vi "Autopatch-v2.4_openlooop.vi"() -> ()   [LabVIEW 2018]
uses:
  <vilib>/userdefined/High Color/IMAQdx.ctl
  <vilib>/DAQmx/write.llb/DAQmx Write (Analog DBL 1Chan 1Samp).vi
  <vilib>/DAQmx/write.llb/DAQmx Write (Analog Wfm 1Chan NSamp).vi
  <vilib>/DAQmx/read.llb/DAQmx Read (Analog Wfm 1Chan NSamp).vi
  <vilib>/Analysis/baseanly.llb/Mean (DBL).vi
  <vilib>/DAQmx/create/channels.llb/DAQmx Create Channel (AO-Voltage-Basic).vi
  <vilib>/DAQmx/miscellaneous.llb/DAQmx Fill In Error Info.vi
  <vilib>/DAQmx/create/channels.llb/DAQmx Create Channel (AI-Voltage-Basic).vi
  <vilib>/DAQmx/configure/timing.llb/DAQmx Timing (Sample Clock).vi
  <vilib>/DAQmx/configure/trigger.llb/DAQmx Start Trigger (Digital Edge).vi
  <vilib>/Waveform/WDTOps.llb/WDT Waveform Duration DBL.vi
  <vilib>/addons/control/pid/pid.llb/PID (DBL).vi
  <vilib>/vision/driver/NI_Vision_Acquisition_Software.lvlib
  <resource>/objmgr/daqmx.rc
  <vilib>/Analysis/NI_AALBase.lvlib
  <vilib>/measure/NI_MABase.lvlib
  <vilib>/vision/NI_Vision_Development_Module.lvlib
  <vilib>/addons/control/pid/NI_PID_pid.lvlib
  <vilib>/Analysis/NI_AALPro.lvlib
panel:
  in  "傅里叶mp285下降步伐":dbl
  in  "下降40倍物镜状态机":u16(ring) items=["下降40倍物镜初始", "下降40倍物镜循环", "下降40倍物镜一段距离", "下降40倍物镜结束", ""]
  in  "气压选择":u16(ring) items=["高正压", "低正压", "大气压", "低负压", "高负压"]
  out "裁剪数组":i32[](array[numeric])
  out "自动接触状态":i32
  in  "没有细胞":bool=TRUE
  out "已发送图像":bool
  in  "发送次数":dbl
  in  "目标细胞位置":bool=TRUE
  out "错误输出 2":errorcluster caption="错误输出"
  out "Matches 2":T1(array[cluster]) {"Bounding Box"."y" format="%.2f"; "Bounding Box"."x" format="%.2f"; "Position"."y" format="%.2f"; "Position"."x" format="%.2f"; "Score" format="%.2f"; "Scale" format="%.2f"; "Angle" format="%.2f"}
  in  "基路径40":path=path "D:/韩宇/程序/CCD/模板40倍.jpg"
  out "傅里叶最大值":dbl
  out "傅里叶数组":bool[](array[boolean])
  in  "傅里叶状态机":u16(ring) items=["傅里叶初始", "傅里叶循环", "傅里叶暂停", "傅里叶结束"]
  out "图像检测到":bool=TRUE
  out "自动封接开始时间":u32
  out "针下降次数":i32
  in  "自动测试":bool
  in  "图像检测":bool
  out "写入的字节":i32
  out "数据输出 3":string
  out "X 3":i32
  out "Y 3":i32
  out "error IO":errorcluster
  out "Y 2":i32
  out "X 2":i32
  in  "开环移动针尖":bool
  in  "傅里叶":bool
  in  "下降物镜":bool
  in  "电极入液":bool
  out "自动接触初始":i32
  in  "枚举":enum16{"200ms", "500ms", "1000ms", ""}(ring)=enum."1000ms"
  out "dX/dt":dbl[](array[numeric])
  in  "下降/向右":bool
  in  "钳制电位":i16(ring) items=["0mv", "-70mv"]
  out "起始破膜时间":u32
  in  "自动破膜":bool
  in  "控制箱刺激ON\n/放大器刺激":bool=TRUE
  in  "自动封接":bool
  in  "保存数据":bool
  out "没匹配到？":bool
  in  "PID gains":T2={"proportional gain (Kc)"=-0.05, "integral time (Ti, min)"=0.0, "derivative time (Td, min)"=0.0} caption="PID增益" {"derivative time (Td, min)" format="%.3f"; "integral time (Ti, min)" format="%.3f"; "proportional gain (Kc)" format="%.3f"}
  in  "PID gains 2":T2={"proportional gain (Kc)"=0.05, "integral time (Ti, min)"=0.0, "derivative time (Td, min)"=0.0} caption="PID增益" {"derivative time (Td, min)" format="%.3f"; "integral time (Ti, min)" format="%.3f"; "proportional gain (Kc)" format="%.3f"}
  in  "下降步伐/um":dbl=1.0
  in  "自动接触":bool
  out "傅里叶求和":sgl(graph)
  in  "针尖移动":bool
  out "目标坐标":i32[](array[numeric])
  in  "针尖模板匹配":bool=TRUE
  in  "基路径20":path=path "D:/韩宇/程序/CCD/针尖水上模板4X.jpg"
  out "Number of Matches":i32
  in  "Minimum Contrast":i32 min=0 max=255 step=1
  in  "Minimum Match Score":sgl=500.0 min=0 max=1000 format="%.2f"
  in  "Number of Matches Requested":i32=1 min=1
  in  "Match Mode":u16(ring) items=["Shift Invariant", "Rotation Invariant"]
  out "针尖坐标":sgl[](array[numeric])
  out "校准的入液阻值":dbl
  out "错误输出 3":errorcluster caption="错误输出"
  out "测量值":dbl
  out "给定值":dbl
  out "输出气压波形图表":cluster{dbl, "低负":dbl}(graph)
  in  "低负":sgl(knob)=-0.45548448
  in  "高负":sgl(knob)=-5.0
  in  "低正":sgl(knob)=0.49642125 scale=0.0..2.0
  in  "高正":sgl(knob)=10.718505 scale=0.0..15.0
  in  "采样率":u32=255
  in  "DevIndex":i32
  in  "Holding Voltage":dbl=-70.0
  out "Negative Peak":dbl
  out "阻值波形图表":dbl(graph)
  out "Resistance(MΩ)":dbl
  out "！":bool
  in  "电压钳/电流钳":u16(ring) items=["Voltage Clamp", "Current Clamp"]
  out "电流信号波形图":waveform(dbl)(graph)
  in  "frequency":dbl=20.0
  in  "Averaging":i32=5
  in  "amplitude":dbl=0.01
  in  "阻值数组":dbl[](array[numeric])
  out "循环时间":u32
  out "Image":T3(plugin-control)
  in  "停止":bool
  in  "Session In":T4="cam1"
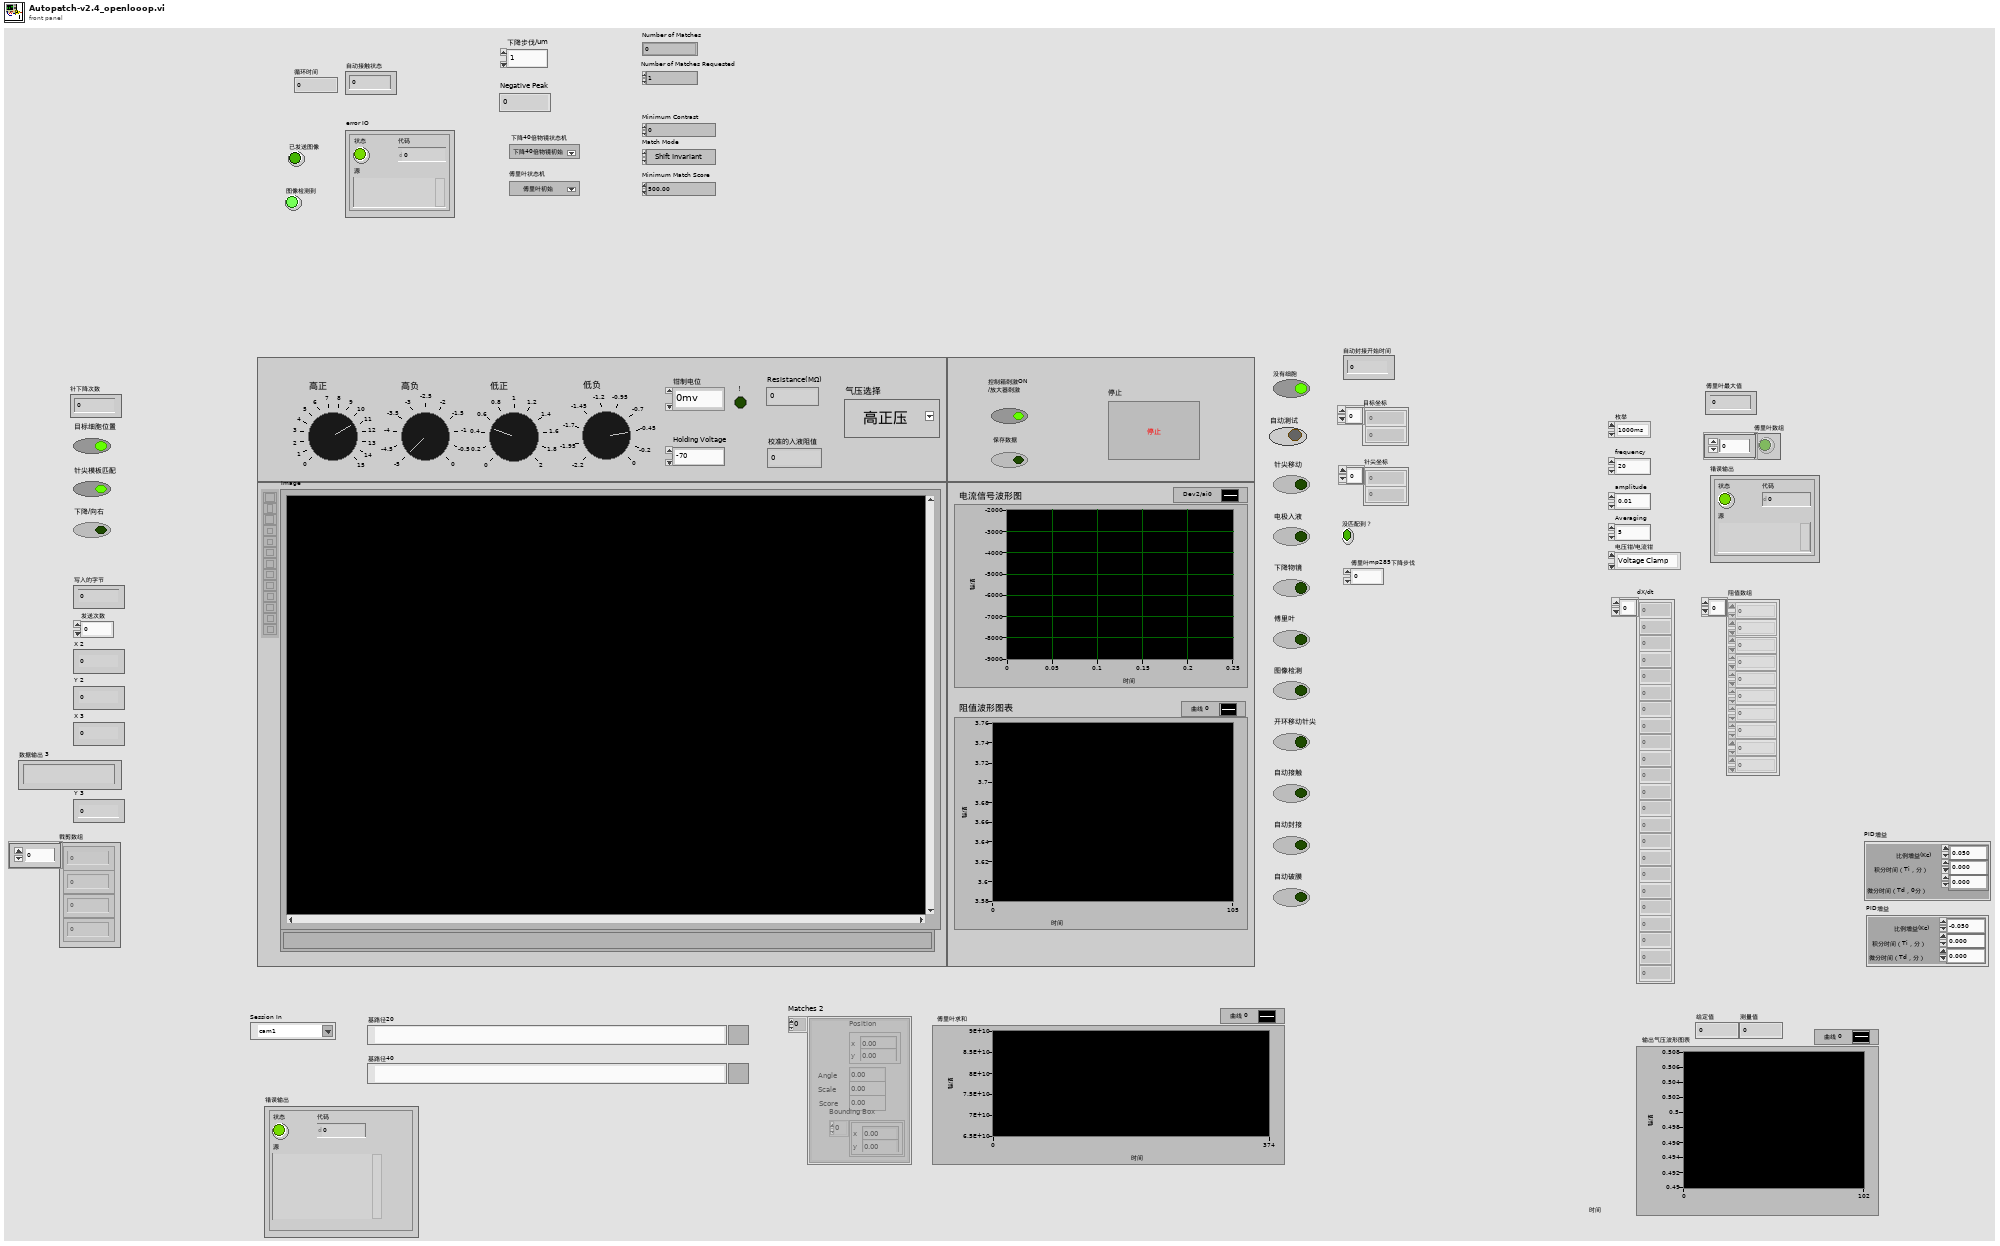
[diagram p1: front panel]
types:
  T1 = cluster{"Position":cluster{"x":sgl, "y":sgl}, "Angle":sgl, "Scale":sgl, "Score":sgl, "Bounding Box":cluster{"x":sgl, "y":sgl}[]}[]
  T2 = cluster{"proportional gain (Kc)":dbl, "integral time (Ti, min)":dbl, "derivative time (Td, min)":dbl}
  T3 = typedef "IMAQ Image.ctl" = refnum<image>
  T4 = typedef "IMAQdx.ctl" = refnum<k21>
  T5 = typedef "Image Type" = u32
  T6 = enum16{"open", "replace", "create", "open or create", "replace or create", "replace or create with confirmation"}
  T7 = cluster{"Averaging":i32, "frequency":dbl, "amplitude":dbl, "Proportion":dbl, "Fs":dbl}
  T8 = enum16{"Sine Wave", "Triangle Wave", "Square Wave", "Sawtooth Wave"}
  T9 = cluster{"Position":cluster{"x":sgl, "y":sgl}, "Angle":sgl, "Scale":sgl, "Score":sgl, "Bounding Box":cluster{"x":sgl, "y":sgl}[]}
  T10 = enum32{"Real", "Imaginary", "Magnitude", "Phase"}
  T11 = cluster{"Global Rectangle":i32[], "Contours":cluster{"Contour Type":u32, "ROI Type":u32, "Points":i32[]}[]}
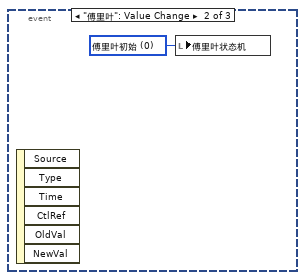
[diagram p7: hidden frame]
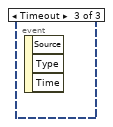
[diagram p8: hidden frame]
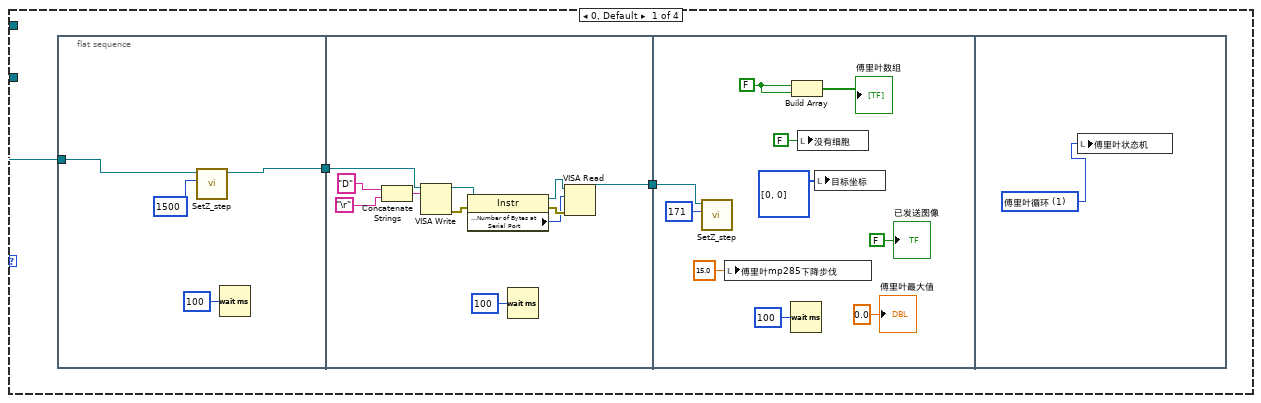
[diagram p12: hidden frame]
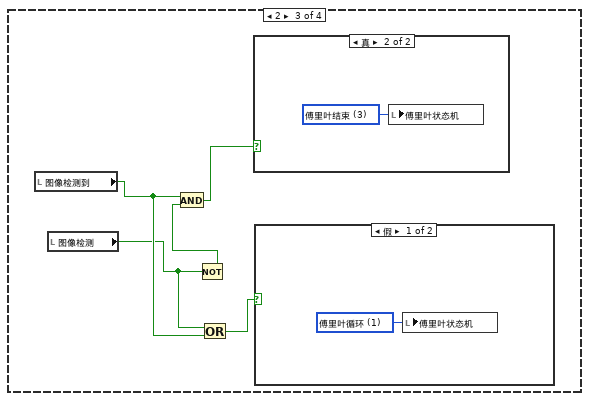
[diagram p16: hidden frame]
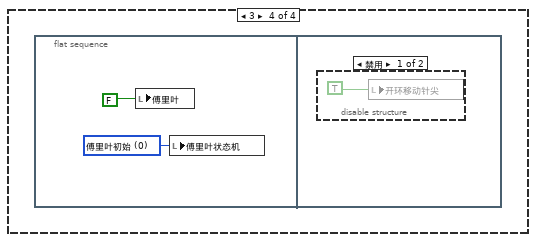
[diagram p19: hidden frame]
diagram:
  w8 = T5 0 items=["Grayscale (U8)", "Grayscale (I16)", "Grayscale (SGL)", "Complex (CSG)", "RGB (U32)", "HSL (U32)", "RGB (U64)", "Grayscale (U16)"] ("Image Type")
  w16 = T5 0 items=["Grayscale (U8)", "Grayscale (I16)", "Grayscale (SGL)", "Complex (CSG)", "RGB (U32)", "HSL (U32)", "RGB (U64)", "Grayscale (U16)"] ("Image Type")
  w23 = T5 3 items=["Grayscale (U8)", "Grayscale (I16)", "Grayscale (SGL)", "Complex (CSG)", "RGB (U32)", "HSL (U32)", "RGB (U64)", "Grayscale (U16)"] ("Image Type")
  w21 = T5 3 items=["Grayscale (U8)", "Grayscale (I16)", "Grayscale (SGL)", "Complex (CSG)", "RGB (U32)", "HSL (U32)", "RGB (U64)", "Grayscale (U16)"] ("Image Type")
  w64 = T5 0 items=["Grayscale (U8)", "Grayscale (I16)", "Grayscale (SGL)", "Complex (CSG)", "RGB (U32)", "HSL (U32)", "RGB (U64)", "Grayscale (U16)"] ("Image Type")
  w77 = FALSE
  # "smacq采集卡初始化"
  # "Mp285"
  # "保存数据"
  n1 = case shown="真" "自动测试" {
    frame False {
    }
    frame True {
      n2 = flat-sequence {
        frame #0 {
          # "每换一次针，\n，请连接网，需要标定初始位置，\n并保存针尖20倍水下模板\n和40倍水下模板，\n以及背景图,调节二值化阈值\n并将针尖移动细胞表面上方,"
          n3 = One Button Dialog(message="请安装玻璃电极并手动移至4倍显微镜视野中央" ("消息")) -> ()  [unwired: 1 in, 1 out]
        }
        frame #1 {
          w138 = u16 1 items=["高正压", "低正压", "大气压", "低负压", "高负压"] ("气压选择")
          n4 = local write "傅里叶"(FALSE ("傅里叶")) -> ()
          n5 = local write "自动接触"(FALSE ("自动接触")) -> ()
          n6 = local write "开环移动针尖"(FALSE ("升Z轴找针")) -> ()
          n7 = local write "针尖移动"(TRUE ("针尖自动移动")) -> ()
          n8 = local write "下降物镜"(FALSE ("自动扫描")) -> ()
          n9 = local write "电极入液"(FALSE ("自动移至工作位置")) -> ()
          n10 = local write "目标坐标"(i32[] [0, 0] ("目标坐标")) -> ()
          n11 = local write "气压选择"(w138) -> ()
        }
      }
    }
  }
  n12 = flat-sequence {
    tunnel: [w148] -> w124
    frame #0 {
      # "选择刺激方式，内部刺激更准"
      n13 = Array Size(array="阻值数组") -> (size(s)=w147:i32)
      n14 = Delete From Array(array="阻值数组", length=w147) -> (array with subset deleted=w145:dbl[])  [unwired: 1 in, 1 out]
      n15 = local write "阻值数组"(w145) -> ()
    }
    frame #1 {
      # "波形个数"
      # "计算电阻波形比例"
      n16 = Bundle("Averaging"="Averaging", "frequency"="frequency", "amplitude"="amplitude", "Proportion"=0.4, "Fs"=20000.0) -> (w148:T7)  [unwired: 1 in]
    }
  }
  n17 = call "OpenDevice.vi"("DevIndex"="DevIndex") -> ("错误输出"=w104:errorcluster, "DevIndex Output"=w102:i32)  [unwired: 9 in]
  n18 = call "SetUSB2AiRange.vi"("错误输入（无错误）"=w104, "Range"=sgl 5.0, "DevIndex"=w102) -> ("错误输出"=w113:errorcluster, "DevIndex Output"=w111:i32)  [unwired: 7 in]
  n19 = call "SetSampleRate.vi"("错误输入（无错误）"=w113, "SampleRate"="采样率", "DevIndex"=w111) -> ("错误输出"=w114:errorcluster, "DevIndex Output"=w112:i32)  [unwired: 7 in]
  n20 = call "SetTrigSource.vi"("错误输入（无错误）"=w114, "TrigSource"=u8 0, "DevIndex"=w112) -> ("错误输出"=w109:errorcluster, "DevIndex Output"=w108:i32)  [unwired: 7 in]
  n21 = call "SetSoftTrig.vi"("错误输入（无错误）"=w109, "Trig"=u8 1, "DevIndex"=w108) -> ("错误输出"=w105:errorcluster, "DevIndex Output"=w103:i32)  [unwired: 7 in]
  n22 = call <vilib>:"IMAQdx Open Camera.vi"("Session In"="Session In") -> ("error out"=w135:errorcluster, "Session Out"=w132:T4)  [unwired: 9 in]
  n23 = disable-structure shown="禁用" {
    disable-tunnel: [w154 _] -> w27
    frame Disabled {
      # "XY移动平台"
      n24 = call "285_Initialize_1.vi"() -> ("VISA资源名称输出"=w154:refnum<visa-resource-name>)  [unwired: 10 in, 1 out]
    }
    frame Enabled {
    }
  }
  n25 = Obtain Queue(element data type=FALSE) -> (queue out=w30:refnum<queue>, error out=w29:errorcluster)  [unwired: 4 in, 1 out]
  n26 = call "InitDA.vi"("错误输入（无错误）"=w105, "DevIndex"=w103) -> ("错误输出"=w99:errorcluster, "DevIndex Output"=w100:i32)  [unwired: 8 in]
  n27 = call <vilib>:"IMAQdx Configure Grab.vi"("error in"=w135, "Session In"=w132) -> ("error out"=w121:errorcluster, "Session Out"=w133:T4)  [unwired: 8 in]
  n28 = call "IMAQ Create"("Image Name"="原图像") -> ("New Image"=w131:T3, "error out"=w119:errorcluster)  [unwired: 4 in]
  n29 = call "IMAQ Create"("Image Name"="灰度图") -> ("New Image"=w125:T3)  [unwired: 4 in, 1 out]
  n30 = call "PRIOR_Initialize.vi"() -> ("VISA资源名称输出"=w4:refnum<visa-resource-name>)  [unwired: 10 in, 1 out]
  n31 = call "285_Initialize.vi"() -> ("VISA资源名称输出"=w28:refnum<visa-resource-name>)  [unwired: 10 in, 1 out]
  n32 = while {
    tunnel: w100 -> [w167]
    tunnel: w30 -> [w206]
    tunnel: w29 -> [w205]
    tunnel: [w160] -> w32
    tunnel: w99 -> [w166]
    tunnel: [w159] -> w31
    stop <- w202 stop-if-true
    # "设置四路气压大小"
    # "事件"
    # "气压控制循环"
    # "气压到电压转换"
    n33 = Dequeue Element(queue=w206, timeout in ms (-1)=1 ("超时毫秒(-1)"), error in (no error)=w205) -> (error out=w203:errorcluster)  [unwired: 3 out]
    n34 = In Range and Coerce(upper limit=sgl 15.0 ("上限"), x="高正", lower limit=sgl 0.0 ("下限")) -> (coerced(x)=w170:sgl)  [unwired: 1 out]
    n35 = In Range and Coerce(upper limit=sgl 0.0 ("上限"), x="高负", lower limit=sgl -5.0 ("下限")) -> (coerced(x)=w174:sgl)  [unwired: 1 out]
    n36 = Unbundle By Name(w203) -> ("status"=w202:bool)
    n37 = Divide(x=w170, y=3) -> (x/y=w191:sgl)
    n38 = Divide(x=w174, y=-1.004) -> (x/y=w187:dbl)
    n39 = In Range and Coerce(upper limit=sgl 2.0 ("上限"), x="低正", lower limit=sgl 0.0 ("下限")) -> (coerced(x)=w178:sgl)  [unwired: 1 out]
    n40 = call "SetDA.vi"("错误输入（无错误）"=w166, "DAVolt"=w191, "DANum"=u8 0, "DevIndex"=w167) -> ("错误输出"=w200:errorcluster, "DevIndex Output"=w201:i32)  [unwired: 6 in]
    n41 = In Range and Coerce(upper limit=sgl 0.0 ("上限"), x="低负", lower limit=sgl -2.2 ("下限")) -> (coerced(x)=w180:sgl)  [unwired: 1 out]
    n42 = call "SetDA.vi"("错误输入（无错误）"=w200, "DAVolt"=w187, "DANum"=u8 1, "DevIndex"=w201) -> ("错误输出"=w199:errorcluster, "DevIndex Output"=w198:i32)  [unwired: 6 in]
    n43 = Multiply(x=w178, y=2.564) -> (x*y=w184:dbl)
    n44 = Multiply(x=w180, y=-2.294) -> (x*y=w185:dbl)
    n45 = call "SetDA.vi"("错误输入（无错误）"=w199, "DAVolt"=w184, "DANum"=u8 2, "DevIndex"=w198) -> ("错误输出"=w196:errorcluster, "DevIndex Output"=w197:i32)  [unwired: 6 in]
    n46 = call "SetDA.vi"("错误输入（无错误）"=w196, "DAVolt"=w185, "DANum"=u8 3, "DevIndex"=w197) -> ("错误输出"=w161:errorcluster, "DevIndex Output"=w162:i32)  [unwired: 6 in]
    n47 = event shown="[1] \"自动封接\": 值改变" {
      selector: _ -> [_ _ _]
      dyn-events: _ -> [_ _ _]
      timeout: 1 -> [_ _ _]
      event Timeout {
        n48 = event-data() -> ()  [unwired: 1 in, 3 out]
      }
      event "自动封接": Value Change {
        # "初始值"
        n49 = event-data() -> ()  [unwired: 1 in, 6 out]
        n50 = Tick Count (ms)() -> (millisecond timer value=w265:u32)
        n51 = local write "自动封接开始时间"(w265) -> ()
        n52 = local write "低负"(-0.66) -> ()
      }
      event "自动破膜": Value Change {
        n53 = event-data() -> ()  [unwired: 1 in, 6 out]
        n54 = Tick Count (ms)() -> (millisecond timer value=→"起始破膜时间":u32)
      }
    }
    n55 = case shown="4" "气压选择" {
      tunnel: w162 -> [w291 w311 w333 w357 w381 w394]
      tunnel: w161 -> [w290 w310 w332 w356 w380 w393]
      tunnel: [w291 w293 w324 w351 w373 w391] -> w160
      tunnel: [w290 w301 w325 w350 w374 w390] -> w159
      tunnel: [w288 w292 w316 w340 w364 w388] -> w163
      frame Default {
        w289 = 0.0
        n56 = Bundle(w289, w289) -> (w288:cluster{dbl, dbl})  [unwired: 1 in]
      }
      frame 0 {
        w308 = TRUE
        w309 = FALSE
        n57 = Build Array(w309, w308, w308, w309, w309, w309, w309, w309) -> (w312:bool[])
        n58 = Boolean Array To Number(Boolean array=w312) -> (number=w315:u32)
        n59 = To Unsigned Byte Integer(number=w315) -> (unsigned 8bit integer=w314:u8)
        n60 = call "StartRead.vi"("错误输入（无错误）"=w310, "DevIndex"=w311) -> ("错误输出"=w306:errorcluster, "DevIndex Output"=w307:i32)  [unwired: 8 in]
        n61 = call "SetDioOut.vi"("错误输入（无错误）"=w306, "DioOut"=w314, "DioChanSel"=u8 255, "DevIndex"=w307) -> ("错误输出"=w302:errorcluster, "DevIndex Output"=w303:i32)  [unwired: 6 in]
        n62 = call "GetAiChans.vi"("错误输入（无错误）"=w302, "Num"=u32 1, "ChanSel"=u16 1, "DevIndex"=w303) -> ("错误输出"=w301:errorcluster, "Ai"=w298:sgl[][], "DevIndex Output"=w293:i32)  [unwired: 4 in, 1 out]
        n63 = Index Array(array=w298, index (row)=0, index (col)=0) -> (element=w295:sgl)
        n64 = local read "高正"() -> (w297:sgl)
        n65 = Multiply(x=w295, y=3) -> (x*y=w294:sgl)
        n66 = Bundle(w294, "高正"=w297) -> (w292:cluster{sgl, "高正":sgl})  [unwired: 1 in]
      }
      frame 4 {
        w331 = TRUE
        w330 = FALSE
        n67 = Build Array(w330, w331, w330, w330, w331, w330, w330, w330) -> (w334:bool[])
        n68 = Boolean Array To Number(Boolean array=w334) -> (number=w339:u32)
        n69 = To Unsigned Byte Integer(number=w339) -> (unsigned 8bit integer=w338:u8)
        n70 = call "StartRead.vi"("错误输入（无错误）"=w332, "DevIndex"=w333) -> ("错误输出"=w335:errorcluster, "DevIndex Output"=w336:i32)  [unwired: 8 in]
        n71 = call "SetDioOut.vi"("错误输入（无错误）"=w335, "DioOut"=w338, "DioChanSel"=u8 255, "DevIndex"=w336) -> ("错误输出"=w326:errorcluster, "DevIndex Output"=w327:i32)  [unwired: 6 in]
        n72 = call "GetAiChans.vi"("错误输入（无错误）"=w326, "Num"=u32 1, "ChanSel"=u16 2, "DevIndex"=w327) -> ("错误输出"=w325:errorcluster, "Ai"=w321:sgl[][], "DevIndex Output"=w324:i32)  [unwired: 4 in, 1 out]
        n73 = Unbundle(w326) -> ()  [unwired: 3 out]
        n74 = Index Array(array=w321, index (row)=0, index (col)=0) -> (element=w319:sgl)
        n75 = local read "高负"() -> (w320:sgl)
        n76 = Multiply(x=w319, y=-1.004) -> (x*y=w317:dbl)
        n77 = Bundle(w317, "高负"=w320) -> (w316:cluster{dbl, "高负":sgl})  [unwired: 1 in]
      }
      frame 1 {
        w342 = FALSE
        n78 = Build Array(w342, w342, w342, TRUE, w342, w342, w342, w342) -> (w358:bool[])
        n79 = Boolean Array To Number(Boolean array=w358) -> (number=w363:u32)
        n80 = To Unsigned Byte Integer(number=w363) -> (unsigned 8bit integer=w362:u8)
        n81 = call "StartRead.vi"("错误输入（无错误）"=w356, "DevIndex"=w357) -> ("错误输出"=w359:errorcluster, "DevIndex Output"=w360:i32)  [unwired: 8 in]
        n82 = call "SetDioOut.vi"("错误输入（无错误）"=w359, "DioOut"=w362, "DioChanSel"=u8 255, "DevIndex"=w360) -> ("错误输出"=w352:errorcluster, "DevIndex Output"=w353:i32)  [unwired: 6 in]
        n83 = call "GetAiChans.vi"("错误输入（无错误）"=w352, "Num"=u32 1, "ChanSel"=u16 4, "DevIndex"=w353) -> ("错误输出"=w350:errorcluster, "Ai"=w347:sgl[][], "DevIndex Output"=w351:i32)  [unwired: 4 in, 1 out]
        n84 = Unbundle(w352) -> ()  [unwired: 3 out]
        n85 = Index Array(array=w347, index (row)=0, index (col)=0) -> (element=w345:sgl)
        n86 = local read "低正"() -> (w346:sgl)
        n87 = Divide(x=w345, y=2.564) -> (x/y=w343:dbl)
        n88 = Bundle(w343, "低正"=w346) -> (w340:cluster{dbl, "低正":sgl})  [unwired: 1 in]
      }
      frame 3 {
        w365 = FALSE
        n89 = call "StartRead.vi"("错误输入（无错误）"=w380, "DevIndex"=w381) -> ("错误输出"=w383:errorcluster, "DevIndex Output"=w384:i32)  [unwired: 8 in]
        n90 = local read "低负"() -> (w369:sgl)
        n91 = Build Array(w365, w365, w365, w365, w365, TRUE, w365, w365) -> (w382:bool[])
        n92 = Boolean Array To Number(Boolean array=w382) -> (number=w387:u32)
        n93 = To Unsigned Byte Integer(number=w387) -> (unsigned 8bit integer=w386:u8)
        n94 = call "SetDioOut.vi"("错误输入（无错误）"=w383, "DioOut"=w386, "DioChanSel"=u8 255, "DevIndex"=w384) -> ("错误输出"=w375:errorcluster, "DevIndex Output"=w376:i32)  [unwired: 6 in]
        n95 = Unbundle(w375) -> ()  [unwired: 3 out]
        n96 = call "GetAiChans.vi"("错误输入（无错误）"=w375, "Num"=u32 1, "ChanSel"=u16 8, "DevIndex"=w376) -> ("错误输出"=w374:errorcluster, "Ai"=w370:sgl[][], "DevIndex Output"=w373:i32)  [unwired: 4 in, 1 out]
        n97 = Index Array(array=w370, index (row)=0, index (col)=0) -> (element=w368:sgl)
        n98 = Divide(x=w368, y=-2.294) -> (x/y=w366:dbl)
        n99 = Bundle(w366, "低负"=w369) -> (w364:cluster{dbl, "低负":sgl})  [unwired: 1 in]
      }
      frame 2 {
        w389 = 0.0
        (unwired) TRUE
        w392 = FALSE
        n100 = call "StartRead.vi"("错误输入（无错误）"=w393, "DevIndex"=w394) -> ("错误输出"=w396:errorcluster, "DevIndex Output"=w397:i32)  [unwired: 8 in]
        n101 = Build Array(w392, w392, w392, w392, w392, w392, w392, w392) -> (w395:bool[])
        n102 = Boolean Array To Number(Boolean array=w395) -> (number=w400:u32)
        n103 = To Unsigned Byte Integer(number=w400) -> (unsigned 8bit integer=w399:u8)
        n104 = call "SetDioOut.vi"("错误输入（无错误）"=w396, "DioOut"=w399, "DioChanSel"=u8 255, "DevIndex"=w397) -> ("错误输出"=w390:errorcluster, "DevIndex Output"=w391:i32)  [unwired: 6 in]
        n105 = Unbundle(w390) -> ()  [unwired: 3 out]
        n106 = Bundle(w389, w389) -> (w388:cluster{dbl, dbl})  [unwired: 1 in]
      }
    }
    "输出气压波形图表" <- w163
    n107 = Unbundle(w163) -> (→"测量值":dbl, "高正"=→"给定值":dbl)
    n108 = case shown="真" "自动封接" {
      frame False {
      }
      frame True {
        w211 = 100.0 ("y")
        w221 = 1300.0 ("y")
        n109 = local read "阻值数组"() -> (w222:dbl[])
        n110 = disable-structure shown="禁用" {
          frame Disabled {
            # "阈值确定？？"
            # "气压微调"
            n111 = local read "阻值数组"() -> (w237:dbl[])
            n112 = call <vilib>:"Derivative x(t).vi"("X"=w237) -> ("dX/dt"=w234:dbl[])  [unwired: 9 in, 1 out]
            "dX/dt" <- w234
            n113 = Index Array(array=w234, index=2 ("索引")) -> (element=w230:dbl)
            n114 = Greater?(x=w230, y=100.0) -> (0:w236:bool)
            n115 = Less?(x=w230, y=10.0) -> (x < y?=w235:bool)
            n116 = case shown="真" w236 {
              frame False {
              }
              frame True {
                n117 = local read "低负"() -> (w245:sgl)
                n118 = Add(x=0.05, y=w245) -> (x+y=w248:dbl)
                n119 = In Range and Coerce(upper limit=0.0, x=w248, lower limit=-1.5) -> (coerced(x)=w244:dbl)  [unwired: 1 out]
                n120 = local write "低负"(w244) -> ()
              }
            }
            n121 = case shown="真" w235 {
              frame False {
              }
              frame True {
                n122 = local read "低负"() -> (w239:sgl)
                n123 = Add(x=-0.05, y=w239) -> (x+y=w242:dbl)
                n124 = In Range and Coerce(upper limit=0.0, x=w242, lower limit=-1.5) -> (coerced(x)=w238:dbl)  [unwired: 1 out]
                n125 = local write "低负"(w238) -> ()
              }
            }
          }
          frame Enabled {
          }
        }
        n126 = Index Array(array=w222, index=0 ("索引")) -> (element=w214:dbl)
        n127 = Index Array(array=w222, index=1 ("索引")) -> (element=w213:dbl)
        n128 = Index Array(array=w222, index=2 ("索引")) -> (element=w212:dbl)
        n129 = Index Array(array=w222, index=3 ("索引")) -> (element=w224:dbl)
        n130 = Index Array(array=w222, index=4 ("索引")) -> (element=w223:dbl)
        n131 = Greater?(x=w214, y=w221) -> (0:w220:bool)
        n132 = Greater?(x=w212, y=w221) -> (0:w218:bool)
        n133 = Greater?(x=w213, y=w221) -> (0:w219:bool)
        n134 = Greater?(x=w224, y=w221) -> (0:w217:bool)
        n135 = Greater?(x=w223, y=w221) -> (0:w216:bool)
        n136 = Compound Arithmetic op=AND ("复合运算")(w220, w219, w218, w217, w216) -> (w215:bool)
        n137 = Greater?(x=w214, y=w211) -> (0:w210:bool)
        n138 = Greater?(x=w213, y=w211) -> (0:w209:bool)
        n139 = Greater?(x=w212, y=w211) -> (0:w208:bool)
        n140 = Compound Arithmetic op=AND ("复合运算")(w210, w209, w208) -> (w207:bool)
        n141 = case shown="假" w207 {
          frame False {
            w250 = i16 0 items=["0mv", "-70mv"] ("钳制电位")
            n142 = local write "钳制电位"(w250) -> ()
          }
          frame True {
            w251 = i16 1 items=["0mv", "-70mv"] ("钳制电位")
            n143 = local write "钳制电位"(w251) -> ()
          }
        }
        n144 = case shown="真" w215 {
          frame True {
            n145 = flat-sequence {
              frame #0 {
                w252 = u16 2 items=["高正压", "低正压", "大气压", "低负压", "高负压"] ("气压选择")
                n146 = local write "气压选择"(w252) -> ()
              }
              frame #1 {
                n147 = Tick Count (ms)() -> (millisecond timer value=w253:u32)
                n148 = local write "起始破膜时间"(w253) -> ()
                n149 = local write "自动破膜"(TRUE) -> ()
                n150 = local write "自动封接"(FALSE) -> ()
                n151 = One Button Dialog(message="已形成G欧封接！" ("消息")) -> ()  [unwired: 1 in, 1 out]
              }
            }
          }
          frame False {
            n152 = flat-sequence {
              frame #0 {
                w257 = u16 3 items=["高正压", "低正压", "大气压", "低负压", "高负压"] ("气压选择")
                n153 = local write "气压选择"(w257) -> ()
              }
              frame #1 {
                n154 = local read "自动封接开始时间"() -> (w261:u32)
                n155 = Tick Count (ms)() -> (millisecond timer value=w262:u32)
                n156 = Subtract(x=w262, y=w261) -> (x-y=w260:u32)
                n157 = Greater?(x=w260, y=u32 200000) -> (0:w258:bool)
                n158 = case shown="真" w258 {
                  frame False {
                  }
                  frame True {
                    n159 = local write "自动封接"(FALSE) -> ()
                    n160 = One Button Dialog(message="自动封接失败！！" ("消息")) -> ()  [unwired: 1 in, 1 out]
                  }
                }
              }
            }
          }
        }
      }
    }
    n161 = case shown="真" "自动破膜" {
      frame False {
      }
      frame True {
        n162 = local read "阻值数组"() -> (w272:dbl[])
        n163 = Index Array(array=w272, index=0 ("索引")) -> (element=w268:dbl)
        n164 = Less?(x=500.0 ("y"), y=w268) -> (x < y?=w270:bool)
        n165 = case shown="真" w270 {
          frame False {
            n166 = local write "自动破膜"(FALSE) -> ()
            n167 = One Button Dialog(message="恭喜你，成功破膜" ("消息")) -> ()  [unwired: 1 in, 1 out]
          }
          frame True {
            n168 = case shown="\"1000ms\"" "枚举" {
              tunnel: [200.0 1000.0 500.0] -> w275
              frame "200ms", Default {
              }
              frame "1000ms" {
              }
              frame "500ms" {
              }
            }
            n169 = Tick Count (ms)() -> (millisecond timer value=w277:u32)
            n170 = local read "起始破膜时间"() -> (w280:u32)
            n171 = Subtract(x=w277, y=w280) -> (x-y=w278:u32)
            n172 = Greater?(x=w275, y=w278) -> (0:w279:bool)
            n173 = case shown="真" w279 {
              frame False {
                n174 = flat-sequence {
                  frame #0 {
                    w284 = u16 2 items=["高正压", "低正压", "大气压", "低负压", "高负压"] ("气压选择")
                    n175 = local write "气压选择"(w284) -> ()
                  }
                  frame #1 {
                    n176 = local write "自动破膜"(FALSE ("自动破膜")) -> ()
                  }
                }
              }
              frame True {
                n177 = flat-sequence {
                  frame #0 {
                    w286 = u16 4 items=["高正压", "低正压", "大气压", "低负压", "高负压"] ("气压选择")
                    n178 = local write "气压选择"(w286) -> ()
                  }
                  frame #1 {
                    n179 = local write "高负"(-5.0) -> ()
                  }
                }
              }
            }
          }
        }
      }
    }
  }
  n180 = call "IMAQ Create"("Image Name"="针尖模板40倍", "Image Type"=w16) -> ("New Image"=w15:T3)  [unwired: 3 in, 1 out]
  n181 = call "IMAQ Create"("Image Name"="针尖模板4倍", "Image Type"=w64) -> ("New Image"=w65:T3)  [unwired: 3 in, 1 out]
  n182 = call "IMAQ ReadFile 2"("File Path"="基路径40", "Image"=w15) -> ("Image Out"=w13:T3)  [unwired: 5 in, 4 out]
  n183 = call "IMAQ ReadFile 2"("File Path"="基路径20", "Image"=w65) -> ("Image Out"=w63:T3)  [unwired: 5 in, 4 out]
  n184 = while {
    tunnel: w124 -> [w409]
    tunnel: [w408] -> w3
    tunnel: w30 -> [w407]
    tunnel: w29 -> [w406]
    stop <- w404 stop-if-true
    # "电流信号循环"
    n185 = Dequeue Element(queue=w407, timeout in ms (-1)=1 ("超时毫秒(-1)"), error in (no error)=w406) -> (error out=w403:errorcluster)  [unwired: 3 out]
    n186 = Unbundle By Name(w403) -> ("status"=w404:bool)
    n187 = flat-sequence {
      tunnel: w409 -> [w428]
      tunnel: [w428] -> w402
      tunnel: [w416] -> w401
      tunnel: [w436] -> w411
      tunnel: [w451] -> w410
      tunnel: w402 -> [w437]
      tunnel: w401 -> [w451]
      tunnel: [w473] -> w415
      tunnel: [w458] -> w414
      tunnel: w411 -> [w453]
      tunnel: w410 -> [w469]
      tunnel: w415 -> [w546]
      tunnel: w414 -> [w547]
      tunnel: w409 -> [w548]
      tunnel: [w545] -> w413
      tunnel: [w537] -> w412
      tunnel: [w590] -> w408
      tunnel: w413 -> [w590]
      tunnel: w412 -> [w588]
      frame #0 {
        n188 = case shown="假" "控制箱刺激ON\n/放大器刺激" {
          tunnel: [0.0 ("data") 5.0 ("data")] -> w425
          frame False {
          }
          frame True {
          }
        }
        n189 = call-poly <vilib>:"DAQmx Create Virtual Channel.vi"("physical channels"=tag "Dev2/ao1") -> ("task out"=w421:refnum<k21>, "error out"=w422:errorcluster)  [unwired: 13 in]
        n190 = call <vilib>:"DAQmx Start Task.vi"("task/channels in"=w421, "error in"=w422) -> ("task out"=w420:refnum<k21>, "error out"=w419:errorcluster)  [unwired: 12 in]
        n191 = call-poly <vilib>:"DAQmx Write.vi"("task/channels in"=w420, "data"=w425, "error in"=w419) -> ("task out"=w418:refnum<k21>, "error out"=w417:errorcluster)  [unwired: 10 in, 1 out]
        n192 = call <vilib>:"DAQmx Stop Task.vi"("task/channels in"=w418, "error in"=w417) -> ("task out"=w424:refnum<k21>, "error out"=w423:errorcluster)  [unwired: 12 in]
        n193 = call <vilib>:"DAQmx Clear Task.vi"("task in"=w424, "error in"=w423) -> ("error out"=w416:errorcluster)  [unwired: 13 in]
      }
      frame #1 {
        n194 = Unbundle By Name(w437) -> ("amplitude"=w443:dbl, "frequency"=w442:dbl, "Fs"=w444:dbl, "Averaging"=w445:i32)
        n195 = Multiply(x=w444, y=w445) -> (x*y=w440:dbl)
        n196 = Multiply(x="钳制电位", y="Holding Voltage") -> (x*y=w433:dbl)
        n197 = Divide(x=w440, y=w442) -> (x/y=w441:dbl)
        n198 = Divide(x=w443, y=2.0) -> (x/y=w447:dbl)
        n199 = Add(x=w433, y=0.5) -> (x+y=w431:dbl)
        n200 = Divide(x=w431, y=1000.0) -> (x/y=w448:dbl)
        n201 = Add(x=w448, y=w447) -> (x+y=w438:dbl)
        n202 = Bundle("Fs"=w444, w441) -> (w446:cluster{"Fs":dbl, dbl})  [unwired: 1 in]
        n203 = call <vilib>:"Basic Function Generator.vi"("offset"=w438, "sampling info"=w446, "signal type"=T8."Square Wave", "amplitude"=w447, "frequency"=w442) -> ("signal out"=w436:waveform(dbl))  [unwired: 4 in, 2 out]
      }
      frame #2 {
        w501 = 10178 items=["有限采样"=10178, "连续采样"=10123, "硬件定时单点"=12522] ("sample mode")
        w502 = tag "OnboardClock" ("source")
        w494 = 10178 items=["有限采样"=10178, "连续采样"=10123, "硬件定时单点"=12522] ("sample mode")
        # "必须要有触发"
        # "This version of StimRecord is for the NI DAQ used in conjunction with the MultiClamp 700b"
        # "multiclamp放大器自己参数"
        # "in V"
        # "in nA"
        n204 = case shown="0, 默认" "电压钳/电流钳" {
          tunnel: [50.0 ("y") 2500000000.0 ("y")] -> w470
          tunnel: [2000.0 ("y") 0.1 ("y")] -> w471
          frame 0, Default {
          }
          frame 1 {
          }
        }
        n205 = Multiply(x=w453, y=w470) -> (x*y=w488:waveform(dbl))
        n206 = call-poly <vilib>:"Waveform Duration.vi"("waveform in"=w453) -> ("duration"=w489:dbl)  [unwired: 8 in, 2 out]
        n207 = Unbundle By Name(w488) -> ("Y"=w457:dbl[], "dt"=w487:dbl)
        n208 = for {
          tunnel: [w516] -> w456 mode=indexing
          tunnel: w457 -> [w510] mode=indexing
          w511 = 10.0 ("t")
          w514 = -10.0 ("t")
          n209 = Greater?(x=w514, y=w510) -> (0:w515:bool)
          n210 = Select(t=w514, s=w515, f=w510) -> (s? t:f=w512:dbl)
          n211 = Less?(x=w511, y=w512) -> (x < y?=w513:bool)
          n212 = Select(t=w511, s=w513, f=w512) -> (s? t:f=w516:dbl)
        }
        n213 = Multiply(x=w489, y=2.0) -> (x*y=w490:dbl)
        n214 = Add(x=w490, y=5.0) -> (x+y=w460:dbl)
        n215 = call-poly <vilib>:"DAQmx Create Virtual Channel.vi"("physical channels"=tag "Dev2/ai0", "error in"=w469) -> ("task out"=w493:refnum<k21>, "error out"=w492:errorcluster)  [unwired: 12 in]
        n216 = call-poly <vilib>:"DAQmx Create Virtual Channel.vi"("physical channels"=tag "Dev2/ao0", "error in"=w469) -> ("task out"=w483:refnum<k21>, "error out"=w482:errorcluster)  [unwired: 12 in]
        n217 = Reciprocal(x=w487) -> (1/x=w495:dbl)
        n218 = Array Size(array=w457) -> (size(s)=w509:i32)
        n219 = call-poly <vilib>:"DAQmx Timing.vi"("task/channels in"=w483, "sample mode"=w501, "samples per channel"=w509, "rate"=w495, "source"=w502, "error in"=w482) -> ("task out"=w468:refnum<k21>, "error out"=w466:errorcluster)  [unwired: 8 in]
        n220 = Bundle By Name(cluster=w488, "Y"=w456) -> (w452:waveform(dbl))
        n221 = call-poly <vilib>:"DAQmx Timing.vi"("task/channels in"=w493, "sample mode"=w494, "samples per channel"=w509, "rate"=w495, "source"=w502, "error in"=w492) -> ("task out"=w497:refnum<k21>, "error out"=w498:errorcluster)  [unwired: 8 in]
        n222 = call-poly <vilib>:"DAQmx Trigger.vi"("task/channels in"=w468, "source"=tag "/Dev2/ai/StartTrigger", "error in"=w466) -> ("task out"=w467:refnum<k21>, "error out"=w465:errorcluster)  [unwired: 11 in]
        n223 = call-poly <vilib>:"DAQmx Write.vi"("task/channels in"=w467, "auto start"=FALSE, "data"=w452, "timeout"=w460, "error in"=w465) -> ("task out"=w486:refnum<k21>, "error out"=w506:errorcluster)  [unwired: 8 in, 1 out]
        n224 = property class="DAQmx定时" props=["SampClk.Rate"](reference=w497, error in=w498) -> (reference out=w499:refnum<k21>)  [unwired: 2 out]
        n225 = call <vilib>:"DAQmx Start Task.vi"("task/channels in"=w486, "error in"=w506) -> ("task out"=w503:refnum<k21>, "error out"=w505:errorcluster)  [unwired: 12 in]
        n226 = call <vilib>:"DAQmx Start Task.vi"("task/channels in"=w499, "error in"=w505) -> ("task out"=w478:refnum<k21>, "error out"=w479:errorcluster)  [unwired: 12 in]
        n227 = call-poly <vilib>:"DAQmx Read.vi"("task/channels in"=w478, "number of samples per channel"=w509, "timeout"=w460, "error in"=w479) -> ("task out"=w464:refnum<k21>, "data"=w491:waveform(dbl), "error out"=w462:errorcluster)  [unwired: 9 in]
        n228 = call <vilib>:"DAQmx Is Task Done.vi"("task/channels in"=w503, "error in"=w505) -> ("task out"=w504:refnum<k21>, "error out"=w507:errorcluster)  [unwired: 11 in, 1 out]
        n229 = call <vilib>:"DAQmx Wait Until Done.vi"("task/channels in"=w504, "timeout (sec)"=w460, "error in"=w507) -> ("task out"=w484:refnum<k21>, "error out"=w485:errorcluster)  [unwired: 11 in]
        n230 = call <vilib>:"DAQmx Wait Until Done.vi"("task/channels in"=w464, "timeout (sec)"=w460, "error in"=w462) -> ("task out"=w463:refnum<k21>, "error out"=w461:errorcluster)  [unwired: 11 in]
        n231 = call <vilib>:"DAQmx Stop Task.vi"("task/channels in"=w484, "error in"=w485) -> ("task out"=w481:refnum<k21>, "error out"=w480:errorcluster)  [unwired: 12 in]
        n232 = Multiply(x=w491, y=w471) -> (x*y=w458:waveform(dbl))
        "电流信号波形图" <- w458
        n233 = call <vilib>:"DAQmx Stop Task.vi"("task/channels in"=w463, "error in"=w461) -> ("task out"=w476:refnum<k21>, "error out"=w477:errorcluster)  [unwired: 12 in]
        n234 = call <vilib>:"DAQmx Clear Task.vi"("task in"=w481, "error in"=w480) -> ("error out"=w508:errorcluster)  [unwired: 13 in]
        n235 = call <vilib>:"DAQmx Clear Task.vi"("task in"=w476, "error in"=w477) -> ("error out"=w475:errorcluster)  [unwired: 13 in]
        n236 = Merge Errors(w508, w475) -> (w473:errorcluster)
        n237 = Build Array(w488, w458) -> ()  [unwired: 1 out]
      }
      frame #3 {
        # "数据读取错误"
        # "阻值读取异常处理"
        # "单位换算不明白"
        # "阻值处理"
        # "Convert Volts/pA into MOhms"
        n238 = call "Filter"("error in (no error)"=w546, "Signal"=w547) -> ("error out"=w549:errorcluster, "Filtered Signal"=w541:dynamicdata)  [unwired: 8 in]
        n239 = call "单频测量"("Signals"=w541) -> ("Frequency"=w540:dynamicdata)  [unwired: 9 in, 1 out]
        n240 = Unbundle By Name(w548) -> ("Fs"=w562:dbl, "frequency"=w561:dbl, "Proportion"=w554:dbl)
        n241 = Unbundle By Name(w548) -> ("Averaging"=w560:i32)
        n242 = call "Convert from Dynamic Data"("Dynamic Data Type"=w541) -> ("Array"=w552:dbl[])  [unwired: 3 in]
        n243 = call "从动态数据转换"("Dynamic Data Type"=w540) -> ("Array"=w539:dbl[])  [unwired: 3 in]
        n244 = call-poly <vilib>:"Mean.vi"("X"=w539) -> ("mean"=w536:dbl)  [unwired: 1 out]
        n245 = Divide(x=w562, y=w561) -> (x/y=w565:dbl)
        n246 = Reshape Array(w552, w560, w565) -> (w564:dbl[][])
        n247 = call-poly <vilib>:"Mean.vi"("X"=w552) -> ("mean"=w553:dbl)  [unwired: 1 out]
        n248 = for {
          N: w560 -> [_]
          tunnel: w564 -> [w576] mode=indexing
          tunnel: w549 -> [w583]
          shift-right: [w584] -> w563
          shift-left: dbl[] [] -> [w585]
          tunnel: [w571] -> w559
          tunnel: [w583] -> w545
          tunnel: w554 -> [w575]
          # "不是整个电流的均值"
          # "波形后半段"
          # "波形前半段"
          n249 = Array Size(array=w576) -> (size(s)=w573:i32)
          n250 = Subtract(x=1.0, y=w575) -> (x-y=w578:dbl)
          n251 = Divide(x=w573, y=2) -> (x/y=w580:dbl)
          n252 = Multiply(x=w580, y=w578) -> (x*y=w577:dbl)
          n253 = Split 1D Array(array=w576, index=w580) -> (first subarray=w572:dbl[], second subarray=w581:dbl[])
          n254 = Split 1D Array(array=w572, index=w577) -> (second subarray=w568:dbl[])  [unwired: 1 out]
          n255 = Split 1D Array(array=w581, index=w577) -> (second subarray=w569:dbl[])  [unwired: 1 out]
          n256 = call-poly <vilib>:"Mean.vi"("X"=w568) -> ("mean"=w570:dbl)  [unwired: 1 out]
          n257 = call-poly <vilib>:"Mean.vi"("X"=w569) -> ("mean"=w571:dbl)  [unwired: 1 out]
          n258 = Subtract(x=w570, y=w571) -> (x-y=w574:dbl)
          n259 = Build Array (concatenate)(w585, w574) -> (w584:dbl[])
        }
        "Negative Peak" <- w559
        n260 = Subtract(x=w536, y=sgl 20.0) -> (x-y=w534:dbl)
        n261 = Array Max & Min(array=w552) -> (min value=w551:dbl)  [unwired: 3 out]
        n262 = Absolute Value(x=w534) -> (abs(x)=w533:dbl)
        n263 = Greater?(x=w533, y=0.05) -> (0:w527:bool)
        "！" <- w527
        n264 = Subtract(x=w553, y=w551) -> (x-y=w550:dbl)
        n265 = Unbundle By Name(w548) -> ("amplitude"=w557:dbl)
        n266 = Multiply(x=w557, y=1000000.0) -> (x*y=w544:dbl)
        n267 = Divide(x=w544, y=w550) -> ()  [unwired: 1 out]
        n268 = call-poly <vilib>:"Mean.vi"("X"=w563) -> ("mean"=w558:dbl)  [unwired: 1 out]
        n269 = local read "Resistance(MΩ)"() -> (w530:dbl)
        n270 = Divide(x=w544, y=w558) -> (x/y=w543:dbl)
        n271 = Multiply(x=w543, y=2.0) -> (x*y=w542:dbl)
        n272 = local read "阻值数组"() -> (w538:dbl[])
        n273 = Less?(x=w530, y=100.0) -> (x < y?=w528:bool)
        n274 = And(x=w528, y=w527) -> (x .and. y?=w526:bool)
        n275 = case shown="假" w526 {
          tunnel: w530 -> [_ w567]
          tunnel: w542 -> [w566 _]
          tunnel: [w566 w567] -> w525
          frame False {
          }
          frame True {
          }
        }
        n276 = In Range and Coerce(upper limit=10000.0 ("上限"), x=w525, lower limit=0.0 ("下限")) -> (coerced(x)=w521:dbl)  [unwired: 1 out]
        "阻值波形图表" <- w521
        "Resistance(MΩ)" <- w521
        n277 = Insert Into Array(array=w538, index=0 ("索引"), new element=w521) -> (w537:dbl[])
        n278 = local write "阻值数组"(w537) -> ()
      }
      frame #4 {
        n279 = Array Size(array=w588) -> (size(s)=w587:i32)
        n280 = Greater?(x=w587, y=10) -> (0:w586:bool)
        n281 = case shown="真" w586 {
          tunnel: w588 -> [_ w593]
          frame False {
          }
          frame True {
            n282 = Delete From Array(array=w593, length=1 ("长度")) -> (array with subset deleted=w591:dbl[])  [unwired: 1 in, 1 out]
            n283 = local write "阻值数组"(w591) -> ()
          }
        }
      }
    }
  }
  n284 = call "IMAQ Create"("Image Name"="", "Image Type"=w8) -> ("New Image"=w11:T3)  [unwired: 3 in, 1 out]
  n285 = call "IMAQ ReadFile 2"("File Path"=path "C:/Users/MPQ/Desktop/2.bmp", "Image"=w11) -> ("Image Out"=w7:T3)  [unwired: 5 in, 4 out]
  n286 = call "IMAQ Create"("Image Name"="") -> ("New Image"=w5:T3)  [unwired: 4 in, 1 out]
  n287 = call "IMAQ ExtractSingleColorPlane"("Image Dst"=w5, "Image Src"=w7) -> ()  [unwired: 8 in, 2 out]
  n288 = call "IMAQ Create"("Image Name"="", "Image Type"=w23) -> ("New Image"=w20:T3)  [unwired: 3 in, 1 out]
  n289 = call "IMAQ Create"("Image Name"="", "Image Type"=w21) -> ("New Image"=w19:T3)  [unwired: 3 in, 1 out]
  n290 = call "IMAQ Create"("Image Name"="unet裁剪") -> ("New Image"=w35:T3)  [unwired: 4 in, 1 out]
  n291 = call "IMAQ Create"("Image Name"="mask图像") -> ("New Image"=w33:T3)  [unwired: 4 in, 1 out]
  n292 = while {
    tunnel: w133 -> [w631]
    tunnel: w131 -> [w630]
    tunnel: [w614] -> w127
    shift-right: [w628] -> _
    shift-left: _ -> [w627]
    tunnel: w125 -> [w626]
    tunnel: [w625] -> w122
    tunnel: w121 -> [w624]
    tunnel: [w623] -> w120
    tunnel: w119 -> [w622]
    tunnel: w30 -> [w621]
    tunnel: [w618] -> w117
    shift-right: [w617] -> w116
    shift-left: w29 -> [w616]
    tunnel: w63 -> [w615]
    tunnel: w35 -> [w613]
    tunnel: w33 -> [w603]
    tunnel: w13 -> [w611]
    tunnel: [w602] -> w123
    stop <- "停止" stop-if-true
    w610 = 0 items=["Red", "Green", "Blue", "Hue", "Saturation", "Luminance", "Value", "Intensity"] ("Color Plane")
    # "图像检测"
    # "图像处理循环"
    n293 = Tick Count (ms)() -> (millisecond timer value=w628:u32)
    n294 = call <vilib>:"IMAQdx Grab2.vi"("error in"=w624, "Image In"=w630, "Session In"=w631) -> ("error out"=w623:errorcluster, "Image Out"=w609:T3, "Session Out"=w614:T4)  [unwired: 5 in, 1 out]
    n295 = Subtract(x=w628, y=w627) -> (x-y=→"循环时间":u32)
    n296 = call "IMAQ ExtractSingleColorPlane"("Color Plane"=w610, "error in (no error)"=w622, "Image Dst"=w626, "Image Src"=w609) -> ("error out"=w625:errorcluster, "Image Dst Out"=w602:T3)  [unwired: 6 in]
    n297 = Enqueue Element(queue=w621, element="停止", timeout in ms (-1)=1 ("超时毫秒(-1)"), error in (no error)=w616) -> (queue out=w618:refnum<queue>, error out=w617:errorcluster)  [unwired: 1 out]
    n298 = local read "针尖移动"() -> (w600:bool)
    n299 = local read "电极入液"() -> (w599:bool)
    n300 = Compound Arithmetic op=OR(w599, "针尖模板匹配", w600) -> ()  [unwired: 1 out]
    n301 = Or(x=w600, y=w599) -> (x .or. y?=w598:bool)
    n302 = Or(x=w598, y="针尖模板匹配") -> (x .or. y?=w596:bool)
    n303 = case shown="真" TRUE {
      tunnel: w615 -> [_ w803]
      tunnel: w602 -> [w797 w806]
      tunnel: [w797 w805] -> w604
      tunnel: w611 -> [_ w801]
      tunnel: w596 -> [_ w799]
      tunnel: [FALSE w798] -> w595
      frame False {
      }
      frame True {
        w808 = u32 1 items=["Frame", "Fill", "Highlight"] ("Drawing Mode (Frame)")
        w817 = u16 0 items=["All", "Shift Information", "Rotation Information"] ("Learn Mode")
        # "真：4倍模板匹配\n假：40倍模板匹配"
        # "目标和针尖坐标获取"
        # "模板匹配针尖"
        n304 = case shown="真" w799 {
          tunnel: [w871 w872] -> w802
          tunnel: w803 -> [_ w872]
          tunnel: w801 -> [w871 _]
          frame False {
          }
          frame True {
          }
        }
        n305 = call "IMAQ Setup Match Pattern 2"("Minimum Contrast"="Minimum Contrast", "Match Mode"="Match Mode") -> ("Match Pattern Setup Data"=w821:string)  [unwired: 8 in, 1 out]
        n306 = call "IMAQ Setup Learn Pattern 2"("Learn Mode"=w817) -> ("Learn Pattern Setup Data"=w816:string)  [unwired: 9 in, 1 out]
        n307 = call "IMAQ Learn Pattern 2"("Learn Pattern Setup Data"=w816, "Image"=w802) -> ("Template Image Out"=w814:T3)  [unwired: 8 in, 1 out]
        n308 = call "IMAQ Match Pattern 2"("Minimum Match Score"="Minimum Match Score", "Number of Matches Requested"="Number of Matches Requested", "Match Pattern Setup Data"=w821, "Template Image"=w814, "Image"=w806) -> ("Number of Matches"=→"Number of Matches":i32, "Matches"=w812:T1)  [unwired: 4 in, 1 out]
        "Matches 2" <- w812
        n309 = Index Array(array=w812, index=0 ("索引")) -> (element=w810:T9)
        n310 = Unbundle(w810) -> ("Score"=w800:sgl)  [unwired: 4 out]
        n311 = Index Array(array=w812, index=0 ("索引")) -> (element=w809:T9)
        n312 = case shown="假" w799 {
          tunnel: w809 -> [w826 w856]
          tunnel: [w823 w854] -> w807
          tunnel: w800 -> [w825 w849]
          tunnel: [w824 w847] -> w798
          frame False {
            w827 = 10.0 ("y")
            # "模板针尖偏移量"
            n313 = Less?(x=w825, y=sgl 500.0) -> (x < y?=w824:bool)
            n314 = Unbundle(w826) -> ("Position"=w834:cluster{"x":sgl, "y":sgl})  [unwired: 4 out]
            n315 = Cluster To Array(cluster=w834) -> (array=w830:sgl[])
            n316 = Equal?(x=w830, y=sgl[] [0.0, 0.0]) -> (x = y?=w832:bool[])
            n317 = And Array Elements(Boolean array=w832) -> (logical AND=w831:bool)
            n318 = case shown="假" w831 {
              tunnel: w830 -> [w846 _]
              frame False {
                n319 = local write "针尖坐标"(w846) -> ()
              }
              frame True {
              }
            }
            n320 = Unbundle(w834) -> ("x"=w843:sgl, "y"=w845:sgl)
            n321 = Add(x=w843, y=sgl 43.0) -> (x+y=w844:sgl)
            n322 = Subtract(x=w845, y=w827) -> (x-y=w837:dbl)
            n323 = Add(x=w845, y=w827) -> (x+y=w836:dbl)
            n324 = Subtract(x=w844, y=w827) -> (x-y=w835:dbl)
            n325 = Add(x=w844, y=w827) -> (x+y=w838:dbl)
            n326 = To Long Integer(number=w837) -> (32bit integer=w840:i32)
            n327 = To Long Integer(number=w836) -> (32bit integer=w841:i32)
            n328 = To Long Integer(number=w835) -> (32bit integer=w839:i32)
            n329 = To Long Integer(number=w838) -> (32bit integer=w842:i32)
            n330 = Bundle(w839, w840, w842, w841) -> (w823:cluster{i32, i32, i32, i32})  [unwired: 1 in]
          }
          frame True {
            w857 = 10.0 ("y")
            n331 = Less?(x=w849, y=sgl 800.0) -> (x < y?=w847:bool)
            n332 = Unbundle(w856) -> ("Position"=w855:cluster{"x":sgl, "y":sgl})  [unwired: 4 out]
            n333 = Cluster To Array(cluster=w855) -> (array=w850:sgl[])
            n334 = Equal?(x=w850, y=sgl[] [0.0, 0.0]) -> (x = y?=w852:bool[])
            n335 = And Array Elements(Boolean array=w852) -> (logical AND=w851:bool)
            n336 = case shown="假" w851 {
              tunnel: w850 -> [w870 _]
              frame False {
                "针尖坐标" <- w870
              }
              frame True {
              }
            }
            n337 = Unbundle(w855) -> ("x"=w866:sgl, "y"=w869:sgl)
            n338 = Add(x=w866, y=sgl 0.0) -> (x+y=w868:sgl)
            n339 = Subtract(x=w869, y=w857) -> (x-y=w860:dbl)
            n340 = Add(x=w869, y=w857) -> (x+y=w859:dbl)
            n341 = Subtract(x=w868, y=w857) -> (x-y=w858:dbl)
            n342 = Add(x=w868, y=w857) -> (x+y=w861:dbl)
            n343 = To Long Integer(number=w860) -> (32bit integer=w863:i32)
            n344 = To Long Integer(number=w859) -> (32bit integer=w864:i32)
            n345 = To Long Integer(number=w858) -> (32bit integer=w862:i32)
            n346 = To Long Integer(number=w861) -> (32bit integer=w865:i32)
            n347 = Bundle(w862, w863, w865, w864) -> (w854:cluster{i32, i32, i32, i32})  [unwired: 1 in]
          }
        }
        n348 = call "IMAQ Overlay Oval"("Color"=u32 6618880, "Drawing Mode (Frame)"=w808, "Bounding Rectangle"=w807, "Image"=w806) -> ("Image Out"=w805:T3)  [unwired: 6 in, 1 out]
      }
    }
    "没匹配到？" <- w595
    n349 = case shown="真" "目标细胞位置" {
      tunnel: [w632 w642] -> w605
      tunnel: w604 -> [w632 w641]
      frame False {
      }
      frame True {
        w636 = 0 ("索引")
        n350 = local read "目标坐标"() -> (w640:i32[])
        n351 = Index Array(array=w640, index=w636) -> (element=w638:i32)
        n352 = Index Array(array=w640, index=1 ("索引")) -> (element=w637:i32)
        n353 = Equal?(x=w638, y=w636) -> (x = y?=w635:bool)
        n354 = Equal?(x=w637, y=w636) -> (x = y?=w634:bool)
        n355 = And(x=w635, y=w634) -> (x .and. y?=w633:bool)
        n356 = case shown="假" w633 {
          tunnel: [w656 w659] -> w642
          tunnel: w641 -> [w655 w659]
          tunnel: w637 -> [w644 _]
          tunnel: w638 -> [w643 _]
          frame False {
            w646 = 10 ("y")
            w657 = u32 1 items=["Frame", "Fill"] ("Drawing Mode (Frame)")
            n357 = Subtract(x=w643, y=w646) -> (x-y=w647:i32)
            n358 = Subtract(x=w644, y=w646) -> (x-y=w649:i32)
            n359 = Add(x=w643, y=w646) -> (x+y=w650:i32)
            n360 = Add(x=w644, y=w646) -> (x+y=w648:i32)
            n361 = To Long Integer(number=w647) -> (32bit integer=w651:i32)
            n362 = To Long Integer(number=w649) -> (32bit integer=w652:i32)
            n363 = To Long Integer(number=w650) -> (32bit integer=w654:i32)
            n364 = To Long Integer(number=w648) -> (32bit integer=w653:i32)
            n365 = Bundle(w651, w652, w654, w653) -> (w645:cluster{i32, i32, i32, i32})  [unwired: 1 in]
            n366 = call "IMAQ Overlay Oval"("Color"=u32 16711680, "Drawing Mode (Frame)"=w657, "Bounding Rectangle"=w645, "Image"=w655) -> ("Image Out"=w656:T3)  [unwired: 6 in, 1 out]
          }
          frame True {
          }
        }
      }
    }
    "Image" <- w605
    n367 = Open/Create/Replace File(file path (use dialog)=path "D:/faster-rcnn.pytorch-pytorch-1.0/data.txt" ("文件路径（使用对话框）")) -> (refnum out=w607:refnum<file>)  [unwired: 5 in, 2 out]
    n368 = case shown="真" "图像检测" {
      tunnel: w613 -> [_ w664]
      tunnel: w607 -> [w660 w663]
      tunnel: [w660 w662] -> w606
      tunnel: w603 -> [_ w661]
      frame False {
      }
      frame True {
        n369 = stacked-sequence {
          tunnel: w664 -> [_ _ _ w700 _ _]
          tunnel: w663 -> [_ _ w672 _ _ _]
          tunnel: [_ _ w671 _ _ _] -> w662
          tunnel: w661 -> [_ _ _ w693 _ _]
          frame #0 {
            n370 = local read "Image"() -> (w666:T3)
            n371 = call-poly "IMAQ Write File 2"("File Path"=path "D:/faster-rcnn.pytorch-pytorch-1.0/temp_img/img.png", "Image"=w666) -> ()  [unwired: 8 in, 2 out]
          }
          frame #1 {
            # "等待rcnn预测"
            n372 = Wait (ms)(milliseconds to wait=u32 1000 ("等待时间（毫秒）")) -> ()  [unwired: 1 out]
          }
          frame #2 {
            w679 = 100 ("y")
            n373 = Set File Position(refnum=w672, from (0:start)=enum16{"start", "end", "current"}."start" ("自（0:起始）")) -> (refnum out=w689:refnum<file>, error out=w691:errorcluster)  [unwired: 2 in]
            n374 = Read from Text File(file (use dialog)=w689, count=1 ("计数"), error in=w691) -> (refnum out=w671:refnum<file>, text=w682:string[], error out=→"错误输出 2":errorcluster)  [unwired: 1 in, 1 out]
            n375 = Index Array(array=w682, index=0 ("索引")) -> (element=w677:string)
            n376 = Match Pattern(string=w677, regular expression="," ("正则表达式")) -> (before substring=w676:string, after substring=w675:string)  [unwired: 1 in, 2 out]
            n377 = Decimal String To Number(string=w676) -> (number=w669:i32)  [unwired: 2 in, 1 out]
            "X 2" <- w669
            n378 = Decimal String To Number(string=w675) -> (number=w683:i32)  [unwired: 2 in, 1 out]
            "Y 2" <- w683
            n379 = Subtract(x=w669, y=w679) -> (x-y=w680:i32)
            n380 = Subtract(x=w683, y=w679) -> (x-y=w686:i32)
            n381 = Add(x=w669, y=w679) -> (x+y=w687:i32)
            n382 = Add(x=w683, y=w679) -> (x+y=w685:i32)
            n383 = To Long Integer(number=w680) -> (32bit integer=w681:i32)
            n384 = To Long Integer(number=w686) -> (32bit integer=w674:i32)
            n385 = To Long Integer(number=w687) -> (32bit integer=w673:i32)
            n386 = To Long Integer(number=w685) -> (32bit integer=w684:i32)
            n387 = Build Array(w681, w674, w673, w684) -> (→"裁剪数组":i32[])
          }
          frame #3 {
            w696 = -1 ("y")
            n388 = local read "Y 2"() -> (w697:i32)
            n389 = local read "X 2"() -> (w694:i32)
            n390 = Equal?(x=w694, y=w696) -> (x = y?=w698:bool)
            n391 = Equal?(x=w697, y=w696) -> (x = y?=w699:bool)
            n392 = Or(x=w698, y=w699) -> (x .or. y?=w695:bool)
            n393 = case shown="假" w695 {
              tunnel: w700 -> [w722 _]
              tunnel: w693 -> [w704 _]
              frame False {
                (unwired) "hello" ("数据输入")
                (unwired) "10.134.224.218" ("名称")
                # "tcp通信"
                # "tcp通信"
                n394 = local read "裁剪数组"() -> (w701:i32[])
                n395 = local read "Image"() -> (w723:T3)
                n396 = call "IMAQ Extract 2"("Optional Rectangle"=w701, "Image Dst"=w722, "Image Src"=w723) -> ("Image Dst Out"=w703:T3)  [unwired: 7 in, 1 out]
                n397 = call "IMAQ Resample"("X Resolution"=128, "Y Resolution"=128, "Image Dst"=w704, "Image Src"=w703) -> ("Image Dst Out"=w702:T3)  [unwired: 6 in, 1 out]
                n398 = call "IMAQ ImageToArray"("Image"=w702) -> ("Image Pixels (U8)"=w718:u8[][])  [unwired: 3 in, 4 out]
                n399 = for {
                  tunnel: w718 -> [w749] mode=indexing
                  tunnel: [w748] -> w720 mode=indexing
                  n400 = for {
                    tunnel: w749 -> [w750] mode=indexing
                    tunnel: [w751] -> w748 mode=indexing
                    n401 = Less?(x=w750, y=u8 10) -> (x < y?=w752:bool)
                    n402 = case shown="假" w752 {
                      tunnel: [w754 w766] -> w751
                      tunnel: w750 -> [w755 w767]
                      frame False {
                        n403 = Less?(x=w755, y=u8 100) -> (x < y?=w756:bool)
                        n404 = case shown="真" w756 {
                          tunnel: w755 -> [w759 w761]
                          tunnel: [w758 w760] -> w754
                          frame False {
                            n405 = Number To Decimal String(number=w759) -> (decimal integer string=w758:string)  [unwired: 1 in]
                          }
                          frame True {
                            n406 = Number To Decimal String(number=w761) -> (decimal integer string=w763:string)  [unwired: 1 in]
                            n407 = Concatenate Strings("0" ("字符串"), w763) -> (w760:string)
                          }
                        }
                      }
                      frame True {
                        n408 = Number To Decimal String(number=w767) -> (decimal integer string=w765:string)  [unwired: 1 in]
                        n409 = Concatenate Strings("00" ("字符串"), w765) -> (w766:string)
                      }
                    }
                  }
                }
                n410 = Add(x="发送次数", y=1.0) -> (x+y=w705:dbl)
                n411 = local write "发送次数"(w705) -> ()
                n412 = Concatenate Strings(w720) -> (w717:string)
                n413 = TCP Open Connection(address="10.134.24.208" ("名称"), remote port or service name=u16 8888 ("远程端口或服务名称")) -> (connection ID=w716:refnum<k5>, error out=w715:errorcluster)  [unwired: 3 in]
                n414 = TCP Write(connection ID=w716, data in=w717, error in (no error)=w715) -> (connection ID out=w713:refnum<k5>, bytes written=→"写入的字节":i32, error out=w714:errorcluster)  [unwired: 1 in]
                n415 = case shown="无错误" w714 {
                  selector: w714 -> [w742 _]
                  tunnel: [w732 errorcluster {"status"=FALSE, "code"=0, "source"=""} ("error IO")] -> w712
                  tunnel: [w734 w746] -> w711
                  tunnel: w713 -> [w731 w746]
                  frame No Error {
                    w728 = 1.5625
                    n416 = TCP Read(connection ID=w731, bytes to read=7 ("读取的字节"), error in (no error)=w742) -> (connection ID out=w734:refnum<k5>, data out=w735:string, error out=w733:errorcluster)  [unwired: 2 in]
                    "数据输出 3" <- w735
                    n417 = case shown="无错误" w733 {
                      selector: w733 -> [w744 _]
                      tunnel: [w744 errorcluster {"status"=FALSE, "code"=0, "source"=""} ("error IO")] -> w732
                      frame No Error {
                      }
                      frame Error {
                      }
                    }
                    n418 = String Subset(string=w735, offset (0)=4 ("偏移量(0)"), length (rest)=3 ("长度（剩余）")) -> (substring=w736:string)
                    n419 = String Subset(string=w735, offset (0)=1 ("偏移量(0)"), length (rest)=3 ("长度（剩余）")) -> (substring=w739:string)
                    n420 = Decimal String To Number(string=w736) -> (number=w725:i32)  [unwired: 2 in, 1 out]
                    n421 = Decimal String To Number(string=w739) -> (number=w724:i32)  [unwired: 2 in, 1 out]
                    n422 = Multiply(x=w725, y=w728) -> (x*y=w729:dbl)
                    n423 = Multiply(x=w724, y=w728) -> (x*y=w730:dbl)
                    n424 = Round To Nearest(number=w729) -> (nearest integer value=→"Y 3":dbl)
                    n425 = Round To Nearest(number=w730) -> (nearest integer value=→"X 3":dbl)
                  }
                  frame Error {
                  }
                }
                "error IO" <- w712
                n426 = TCP Close Connection(connection ID=w711, error in (no error)=w712) -> ()  [unwired: 1 in, 2 out]
              }
              frame True {
              }
            }
          }
          frame #4 {
            w770 = -1 ("y")
            n427 = local read "X 3"() -> (w781:i32)
            n428 = local read "Y 3"() -> (w779:i32)
            n429 = local read "X 2"() -> (w774:i32)
            n430 = local read "Y 2"() -> (w773:i32)
            n431 = Equal?(x=w774, y=w770) -> (x = y?=w772:bool)
            n432 = Equal?(x=w773, y=w770) -> (x = y?=w771:bool)
            n433 = Equal?(x=w781, y=0) -> (x = y?=w777:bool)
            n434 = Equal?(x=w779, y=0) -> (x = y?=w776:bool)
            n435 = Or(x=w772, y=w771) -> (x .or. y?=w769:bool)
            n436 = And(x=w777, y=w776) -> (x .and. y?=w775:bool)
            n437 = Or(x=w775, y=w769) -> (x .or. y?=w768:bool)
            n438 = case shown="假" w768 {
              frame False {
                n439 = flat-sequence {
                  frame #0 {
                    "图像检测到" <- TRUE
                  }
                  frame #1 {
                    n440 = local write "图像检测"(FALSE) -> ()
                  }
                }
                n441 = local read "X 2"() -> (w792:i32)
                n442 = local read "X 3"() -> (w791:i32)
                n443 = local read "Y 2"() -> (w790:i32)
                n444 = local read "Y 3"() -> (w789:i32)
                n445 = Add(x=w792, y=w791) -> (x+y=w786:i32)
                n446 = Add(x=w790, y=w789) -> (x+y=w785:i32)
                n447 = Subtract(x=w786, y=100) -> (x-y=w783:i32)
                n448 = Subtract(x=w785, y=100) -> (x-y=w782:i32)
                n449 = Build Array(w783, w782) -> (w784:i32[])
                n450 = local write "目标坐标"(w784) -> ()
              }
              frame True {
              }
            }
          }
          frame #5 {
            n451 = local write "图像检测"(FALSE) -> ()
          }
        }
      }
    }
    n452 = Close File(refnum=w606) -> ()  [unwired: 1 in, 2 out]
  }
  n453 = call "SetDA.vi"("错误输入（无错误）"=w31, "DevIndex"=w32) -> ("错误输出"=w88:errorcluster, "DevIndex Output"=w89:i32)  [unwired: 8 in]
  n454 = call "SetDA.vi"("错误输入（无错误）"=w88, "DAVolt"=0.0, "DANum"=u8 1, "DevIndex"=w89) -> ("错误输出"=w87:errorcluster, "DevIndex Output"=w86:i32)  [unwired: 6 in]
  n455 = Build Array(w77, w77, w77, w77, w77, w77, w77, w77) -> (w75:bool[])
  n456 = call "SetDA.vi"("错误输入（无错误）"=w87, "DAVolt"=0.0, "DANum"=u8 2, "DevIndex"=w86) -> ("错误输出"=w84:errorcluster, "DevIndex Output"=w85:i32)  [unwired: 6 in]
  n457 = Boolean Array To Number(Boolean array=w75) -> (number=w76:u32)
  n458 = call "SetDA.vi"("错误输入（无错误）"=w84, "DAVolt"=0.0, "DANum"=u8 3, "DevIndex"=w85) -> ("错误输出"=w71:errorcluster, "DevIndex Output"=w72:i32)  [unwired: 6 in]
  n459 = To Unsigned Byte Integer(number=w76) -> (unsigned 8bit integer=w74:u8)
  n460 = call "SetDioOut.vi"("错误输入（无错误）"=w71, "DioOut"=w74, "DioChanSel"=u8 255, "DevIndex"=w72) -> ("错误输出"=w70:errorcluster, "DevIndex Output"=w69:i32)  [unwired: 6 in]
  n461 = call "StopRead.vi"("错误输入（无错误）"=w70, "DevIndex"=w69) -> ("错误输出"=w95:errorcluster, "DevIndex Output"=w96:i32)  [unwired: 8 in]
  n462 = call "SetSoftTrig.vi"("错误输入（无错误）"=w95, "Trig"=u8 0, "DevIndex"=w96) -> ("错误输出"=w94:errorcluster, "DevIndex Output"=w92:i32)  [unwired: 7 in]
  n463 = call "ClearTrigger.vi"("错误输入（无错误）"=w94, "DevIndex"=w92) -> ("错误输出"=w93:errorcluster, "DevIndex Output"=w91:i32)  [unwired: 8 in]
  n464 = call "ClearBufs.vi"("错误输入（无错误）"=w93, "DevIndex"=w91) -> ("错误输出"=w97:errorcluster, "DevIndex Output"=w98:i32)  [unwired: 8 in]
  n465 = call "CloseDevice.vi"("错误输入（无错误）"=w97, "DevIndex"=w98) -> ("错误输出"=w61:errorcluster)  [unwired: 8 in, 1 out]
  n466 = Merge Errors(w3, w61) -> (w2:errorcluster)
  n467 = Get Date/Time String(date format (0)=enum16{"short", "long", "abbreviated"}."long" ("日期格式(0)"), want seconds? (F)=TRUE ("需要秒？(F)")) -> (date string=w59:string, time string=w44:string)  [unwired: 1 in]
  n468 = String Subset(string=w44, offset (0)=6 ("偏移量(0)")) -> (substring=w42:string)  [unwired: 1 in]
  n469 = String Subset(string=w44, offset (0)=3 ("偏移量(0)"), length (rest)=2 ("长度（剩余）")) -> (substring=w54:string)
  n470 = String Subset(string=w44, length (rest)=2 ("长度（剩余）")) -> (substring=w56:string)  [unwired: 1 in]
  n471 = Concatenate Strings(w56, "时" ("字符串"), w54, "分" ("字符串"), w42, "秒" ("字符串")) -> (w55:string)
  n472 = Concatenate Strings(w59, w55) -> (w38:string)
  n473 = call "IMAQ Dispose"("Image"=w123, "error in (no error)"=w122) -> ("error out"=w128:errorcluster)  [unwired: 4 in]
  n474 = call <vilib>:"IMAQdx Close Camera.vi"("error in"=w120, "Session In"=w127) -> ("error out"=w129:errorcluster)  [unwired: 9 in]
  n475 = Build Path(base path=path "D:/韩宇/实验/数据" ("文件路径（使用对话框）"), name or relative path=w38) -> (appended path=w52:path)
  n476 = Release Queue(queue=w117, error in (no error)=w116) -> (error out=w68:errorcluster)  [unwired: 1 in, 2 out]
  n477 = Create Folder(path (use dialog)=w52) -> (created path=w47:path)  [unwired: 2 in, 2 out]
  n478 = Merge Errors(w128, w129, w68, w2) -> (→"错误输出 3":errorcluster)
  n479 = Build Path(base path=w47, name or relative path="data.txt" ("字符串")) -> (appended path=w49:path)
  n480 = Open/Create/Replace File(file path (use dialog)=w49, operation (0:open)=T6."open or create" ("操作(0:open)")) -> (refnum out=w48:refnum<file>)  [unwired: 4 in, 2 out]
  n481 = while {
    tunnel: w28 -> [w875]
    tunnel: w29 -> [w900]
    tunnel: w30 -> [w899]
    tunnel: w48 -> [w896]
    tunnel: w47 -> [w895]
    tunnel: [w892] -> w46
    tunnel: w27 -> [_]
    tunnel: w4 -> [w883]
    tunnel: [w891] -> w26
    tunnel: w4 -> [w884]
    tunnel: w20 -> [w888]
    tunnel: w19 -> [w887]
    tunnel: [w888] -> w18
    tunnel: [w887] -> w17
    tunnel: w4 -> [w879]
    i -> [w894]
    stop <- w901 stop-if-true
    # "Mp285A控制循环"
    n482 = Dequeue Element(queue=w899, timeout in ms (-1)=1 ("超时毫秒(-1)"), error in (no error)=w900) -> (error out=w902:errorcluster)  [unwired: 3 out]
    n483 = Unbundle By Name(w902) -> ("status"=w901:bool)
    n484 = event shown="[0] \"自动接触\": 值改变" {
      selector: _ -> [_ _ _]
      dyn-events: _ -> [_ _ _]
      timeout: 1 -> [_ _ _]
      event "自动接触": Value Change {
        # "事件结构有问题"
        n485 = event-data() -> ()  [unwired: 1 in, 6 out]
        n486 = local read "Resistance(MΩ)"() -> (w915:dbl)
        n487 = Greater?(x=w915, y=15.0) -> (0:w912:bool)
        n488 = Less?(x=w915, y=3.0) -> (x < y?=w911:bool)
        n489 = Or(x=w912, y=w911) -> (x .or. y?=w910:bool)
        n490 = local write "校准的入液阻值"(w915) -> ()
        n491 = case shown="真" w910 {
          frame False {
          }
          frame True {
            n492 = local write "自动接触"(FALSE) -> ()
            n493 = One Button Dialog(message="针尖异常" ("消息")) -> ()  [unwired: 1 in, 1 out]
          }
        }
        "自动接触初始" <- 0
        "针下降次数" <- 0 ("针下降次数")
      }
      event "傅里叶": Value Change {
        w920 = u16 0 items=["傅里叶初始", "傅里叶循环", "傅里叶暂停", "傅里叶结束"] ("傅里叶状态机")
        n494 = event-data() -> ()  [unwired: 1 in, 6 out]
        n495 = local write "傅里叶状态机"(w920) -> ()
      }
      event Timeout {
        n496 = event-data() -> ()  [unwired: 1 in, 3 out]
      }
    }
    n497 = case shown="真" "电极入液" {
      tunnel: w875 -> [_ w1091]
      frame False {
      }
      frame True {
        n498 = local read "Resistance(MΩ)"() -> (w1090:dbl)
        n499 = Less?(x=w1090, y=1.0) -> (x < y?=w1094:bool)
        n500 = Greater?(x=w1090, y=100.0) -> (0:w1093:bool)
        n501 = Or(x=w1094, y=w1093) -> (x .or. y?=w1092:bool)
        n502 = case shown="假" w1092 {
          tunnel: w1091 -> [w1097 w1117]
          frame False {
            n503 = stacked-sequence {
              tunnel: w1097 -> [_ _ _ w1103]
              frame #0 {
                w1098 = u16 0 items=["高正压", "低正压", "大气压", "低负压", "高负压"] ("气压选择")
                n504 = local write "电极入液"(FALSE ("电极入液")) -> ()
                n505 = local write "气压选择"(w1098) -> ()
              }
              frame #1 {
                n506 = Wait (ms)(milliseconds to wait=u32 1000 ("等待时间（毫秒）")) -> ()  [unwired: 1 out]
              }
              frame #2 {
                w1102 = u16 1 items=["高正压", "低正压", "大气压", "低负压", "高负压"] ("气压选择")
                n507 = Wait (ms)(milliseconds to wait=u32 1000 ("等待时间（毫秒）")) -> ()  [unwired: 1 out]
                n508 = local write "气压选择"(w1102) -> ()
              }
              frame #3 {
                n509 = local read "Resistance(MΩ)"() -> (w1108:dbl)
                n510 = Less?(x=w1108, y=3.0) -> (x < y?=w1106:bool)
                n511 = Greater?(x=w1108, y=9.0) -> (0:w1105:bool)
                n512 = And(x=w1106, y=w1105) -> (x .and. y?=w1104:bool)
                n513 = case shown="假" w1104 {
                  tunnel: w1103 -> [w1112 _]
                  frame False {
                    w1110 = u16 0 items=["下降40倍物镜初始", "下降40倍物镜循环", "下降40倍物镜一段距离", "下降40倍物镜结束", ""] ("下降40倍物镜状态机")
                    n514 = local write "下降40倍物镜状态机"(w1110) -> ()
                    n515 = local write "下降物镜"(TRUE) -> ()
                    n516 = call "285_RelMove.vi"("VISA资源名称"=w1112, "Z 2"=1000.0, "Y 2"=0.0, "X 2"=0.0) -> ()  [unwired: 2 in, 6 out]
                  }
                  frame True {
                    n517 = One Button Dialog(message="针尖异常" ("消息")) -> ()  [unwired: 1 in, 1 out]
                  }
                }
              }
            }
          }
          frame True {
            n518 = call "285_RelMove.vi"("VISA资源名称"=w1117, "Z 2"=30.0, "Y 2"=0.0, "X 2"=0.0) -> ()  [unwired: 2 in, 6 out]
          }
        }
      }
    }
    n519 = local read "针尖坐标"() -> (w890:sgl[])
    n520 = case shown="真" "下降物镜" {
      tunnel: w879 -> [_ w1066]
      frame False {
      }
      frame True {
        n521 = case shown="0, 默认" "下降40倍物镜状态机" {
          tunnel: w1066 -> [w1069 w1072 _]
          frame 0, Default {
            w1071 = u16 1 items=["下降40倍物镜初始", "下降40倍物镜循环", "下降40倍物镜结束", ""] ("下降40倍物镜状态机")
            n522 = call "SetZ_step.vi"("step"=5, "VISA资源名称"=w1069) -> ()  [unwired: 8 in, 2 out]
            n523 = local write "下降40倍物镜状态机"(w1071) -> ()
            n524 = One Button Dialog(message="请更换40倍物镜，\n并将水镜刚好置于水面\n再加水，调整光强" ("消息")) -> ()  [unwired: 1 in, 1 out]
          }
          frame 1 {
            n525 = flat-sequence {
              tunnel: w1072 -> [w1073]
              frame #0 {
                n526 = Concatenate Strings("D" ("写入缓冲区"), "\r") -> (w1081:string)
                n527 = VISA Write ("VISA写入")(VISA resource name=w1073, write buffer=w1081) -> (VISA resource name out=w1078:refnum<visa-resource-name>, error out=w1077:errorcluster)  [unwired: 1 in, 1 out]
                n528 = property class="Instr"(reference=w1078, error in=w1077) -> (reference out=w1080:refnum<visa-resource-name>, error out=w1076:errorcluster, "Serial Settings:Number of Bytes at Serial Port"=w1079:u32)
                n529 = VISA Read(VISA resource name=w1080, byte count=w1079, error in (no error)=w1076) -> ()  [unwired: 4 out]
              }
              frame #1 {
                n530 = Wait (ms)(milliseconds to wait=u32 100 ("等待时间（毫秒）")) -> ()  [unwired: 1 out]
              }
              frame #2 {
                n531 = local read "没匹配到？"() -> (w1083:bool)
                n532 = case shown="假" w1083 {
                  frame False {
                    w1085 = u16 2 items=["下降40倍物镜初始", "下降40倍物镜循环", "下降40倍物镜一段距离", "下降40倍物镜结束", ""] ("下降40倍物镜状态机")
                    n533 = local write "下降40倍物镜状态机"(w1085) -> ()
                    n534 = Wait (ms)(milliseconds to wait=u32 1000 ("等待时间（毫秒）")) -> ()  [unwired: 1 out]
                  }
                  frame True {
                  }
                }
              }
            }
          }
          frame 2 {
            w1086 = u16 0 items=["下降40倍物镜初始", "下降40倍物镜循环", "下降40倍物镜一段距离", "下降40倍物镜结束", ""] ("下降40倍物镜状态机")
            w1089 = u16 0 items=["傅里叶初始", "傅里叶循环", "傅里叶暂停", "傅里叶结束"] ("傅里叶状态机")
            n535 = local write "下降物镜"(FALSE) -> ()
            n536 = local write "傅里叶"(TRUE ("针尖粗对焦")) -> ()
            n537 = local write "傅里叶状态机"(w1089) -> ()
            n538 = local write "下降40倍物镜状态机"(w1086) -> ()
          }
        }
      }
    }
    n539 = case shown="真" "针尖移动" {
      tunnel: [w1158 w1170] -> w874
      tunnel: sgl[] [1685.0, 1364.0] ("针尖坐标") -> [_ w1172]
      tunnel: w890 -> [_ w1165]
      tunnel: 2000.0 ("y") -> [_ w1160]
      tunnel: w875 -> [w1158 w1159]
      frame False {
      }
      frame True {
        # "模板针尖偏移量"
        # "PID控制针尖移动"
        # "可以直接用pid模块"
        n540 = Index Array(array=w1165, index=1 ("索引")) -> (element=w1162:sgl)
        n541 = Index Array(array=w1165, index=0 ("索引")) -> (element=w1161:sgl)
        n542 = Index Array(array=w1172, index=1 ("索引")) -> (element=w1181:sgl)
        n543 = Index Array(array=w1172, index=0 ("索引")) -> (element=w1182:sgl)
        n544 = Subtract(x=w1181, y=w1162) -> (x-y=w1177:sgl)
        n545 = Bundle("x"=w1162, "x"=w1181) -> ()  [unwired: 1 in, 1 out]
        n546 = Add(x=sgl 0.0 ("y"), y=w1161) -> (x+y=w1166:sgl)
        n547 = Subtract(x=w1182, y=w1166) -> (x-y=w1178:sgl)
        n548 = call-poly <vilib>:"PID.vi"("PID gains"="PID gains", "process variable"=w1166, "setpoint"=w1182) -> ("output"=w1168:dbl)  [unwired: 7 in, 1 out]
        n549 = call-poly <vilib>:"PID.vi"("PID gains"="PID gains 2", "process variable"=w1162, "setpoint"=w1181) -> ("output"=w1169:dbl)  [unwired: 7 in, 1 out]
        n550 = Bundle("x"=w1161, "x"=w1182) -> ()  [unwired: 1 in, 1 out]
        n551 = Square(x=w1178) -> (x^2=w1176:sgl)
        n552 = Square(x=w1177) -> (x^2=w1175:sgl)
        n553 = Add(x=w1176, y=w1175) -> (x+y=w1171:sgl)
        n554 = Greater?(x=w1171, y=w1160) -> (0:w1183:bool)
        n555 = case shown="真" w1183 {
          tunnel: [w1184 w1190] -> w1170
          tunnel: w1168 -> [_ w1189]
          tunnel: w1169 -> [_ w1188]
          tunnel: w1159 -> [w1184 w1187]
          frame False {
            n556 = local write "针尖移动"(FALSE ("针尖自动移动")) -> ()
            n557 = local write "电极入液"(TRUE ("手动换物镜")) -> ()
          }
          frame True {
            # "阈值范围需要调整，太大针尖检测不出来，太小程序会出现bug'"
            n558 = flat-sequence {
              tunnel: [w1197] -> w1190
              tunnel: w1189 -> [w1193]
              tunnel: w1188 -> [w1192]
              tunnel: w1187 -> [w1191]
              frame #0 {
                # "小距离285不动了？？？"
                # "x位置p负号原因是设备转换后的"
                n559 = To Byte Integer(number=w1192) -> (8bit integer=w1196:i8)
                n560 = To Byte Integer(number=w1193) -> (8bit integer=w1195:i8)
                n561 = In Range and Coerce(upper limit=30.0 ("上限"), x=w1196, lower limit=-30.0 ("上限")) -> (coerced(x)=w1200:dbl)  [unwired: 1 out]
                n562 = In Range and Coerce(upper limit=30.0 ("上限"), x=w1195, lower limit=-30.0 ("上限")) -> (coerced(x)=w1194:dbl)  [unwired: 1 out]
                n563 = call "285_RelMove.vi"("VISA资源名称"=w1191, "Z 2"=0.0 ("Z"), "Y 2"=w1200, "X 2"=w1194) -> ("VISA resource name out 2"=w1197:refnum<visa-resource-name>)  [unwired: 2 in, 5 out]
              }
            }
          }
        }
      }
    }
    n564 = case shown="真" "傅里叶" {
      tunnel: w883 -> [_ w946]
      tunnel: w888 -> [_ w945]
      tunnel: w887 -> [_ w944]
      tunnel: w874 -> [_ w943]
      frame False {
      }
      frame True {
        n565 = case shown="1" "傅里叶状态机" {
          tunnel: w946 -> [w950 w985 _ _]
          tunnel: w945 -> [_ w980 _ _]
          tunnel: w944 -> [_ w979 _ _]
          tunnel: w943 -> [_ w977 _ _]
          frame 0, Default {
            n566 = flat-sequence {
              tunnel: w950 -> [w953]
              tunnel: [w952] -> w948
              tunnel: [w956] -> w949
              tunnel: w948 -> [w957]
              tunnel: w949 -> [w968]
              frame #0 {
                n567 = call "SetZ_step.vi"("step"=1500, "VISA资源名称"=w953) -> ("VISA资源名称输出"=w952:refnum<visa-resource-name>)  [unwired: 8 in, 1 out]
                n568 = Wait (ms)(milliseconds to wait=u32 100 ("等待时间（毫秒）")) -> ()  [unwired: 1 out]
              }
              frame #1 {
                n569 = Concatenate Strings("D" ("写入缓冲区"), "\r") -> (w960:string)
                n570 = VISA Write ("VISA写入")(VISA resource name=w957, write buffer=w960) -> (VISA resource name out=w963:refnum<visa-resource-name>, error out=w964:errorcluster)  [unwired: 1 in, 1 out]
                n571 = property class="Instr"(reference=w963, error in=w964) -> (reference out=w961:refnum<visa-resource-name>, error out=w965:errorcluster, "Serial Settings:Number of Bytes at Serial Port"=w962:u32)
                n572 = Wait (ms)(milliseconds to wait=u32 100 ("等待时间（毫秒）")) -> ()  [unwired: 1 out]
                n573 = VISA Read(VISA resource name=w961, byte count=w962, error in (no error)=w965) -> (VISA resource name out=w956:refnum<visa-resource-name>)  [unwired: 3 out]
              }
              frame #2 {
                w974 = FALSE
                n574 = call "SetZ_step.vi"("step"=171, "VISA资源名称"=w968) -> ()  [unwired: 8 in, 2 out]
                n575 = local write "傅里叶mp285下降步伐"(15.0 ("傅里叶mp285下降步伐")) -> ()
                n576 = Wait (ms)(milliseconds to wait=u32 100 ("等待时间（毫秒）")) -> ()  [unwired: 1 out]
                n577 = Build Array(w974, w974) -> (→"傅里叶数组":bool[])
                n578 = local write "没有细胞"(FALSE ("没有细胞")) -> ()
                n579 = local write "目标坐标"(i32[] [0, 0] ("目标坐标")) -> ()
                "傅里叶最大值" <- 0.0
                "已发送图像" <- FALSE ("已发送图像")
              }
              frame #3 {
                w976 = u16 1 items=["傅里叶初始", "傅里叶循环", "傅里叶暂停", "傅里叶结束"] ("傅里叶状态机")
                n580 = local write "傅里叶状态机"(w976) -> ()
              }
            }
          }
          frame 1 {
            n581 = flat-sequence {
              tunnel: w985 -> [w992]
              tunnel: [w991] -> w984
              tunnel: w977 -> [w988]
              tunnel: w984 -> [w1002]
              tunnel: [w1001] -> w978
              tunnel: [w1009] -> w983
              tunnel: w980 -> [w1030]
              tunnel: w979 -> [w1031]
              tunnel: w978 -> [w1012]
              tunnel: w983 -> [w1037]
              tunnel: [w1039] -> w982
              tunnel: [w1038] -> w981
              tunnel: w982 -> [w1048]
              tunnel: w981 -> [w1047]
              frame #0 {
                n582 = Concatenate Strings("D" ("写入缓冲区"), "\r") -> (w1000:string)
                n583 = VISA Write ("VISA写入")(VISA resource name=w992, write buffer=w1000) -> (VISA resource name out=w995:refnum<visa-resource-name>, error out=w997:errorcluster)  [unwired: 1 in, 1 out]
                n584 = Wait (ms)(milliseconds to wait=u32 100 ("等待时间（毫秒）")) -> ()  [unwired: 1 out]
                n585 = call "285_RelMove.vi"("VISA资源名称"=w988, "Z 2"="傅里叶mp285下降步伐", "Y 2"=0.0, "X 2"=0.0) -> ()  [unwired: 2 in, 6 out]
                n586 = property class="Instr"(reference=w995, error in=w997) -> (reference out=w998:refnum<visa-resource-name>, error out=w999:errorcluster, "Serial Settings:Number of Bytes at Serial Port"=w996:u32)
                n587 = VISA Read(VISA resource name=w998, byte count=w996, error in (no error)=w999) -> (VISA resource name out=w991:refnum<visa-resource-name>)  [unwired: 3 out]
              }
              frame #1 {
                n588 = VISA Flush I/O Buffer(VISA resource name=w1002) -> (VISA resource name out=w1001:refnum<visa-resource-name>)  [unwired: 2 in, 1 out]
                n589 = Wait (ms)(milliseconds to wait=u32 50 ("等待时间（毫秒）")) -> ()  [unwired: 1 out]
              }
              frame #2 {
                n590 = local read "Image"() -> (w1015:T3)
                n591 = call "IMAQ ImageToArray"("Image"=w1015) -> ("error out"=w1022:errorcluster, "Image Pixels (U8)"=w1014:u8[][])  [unwired: 3 in, 3 out]
                n592 = call "IMAQ ArrayToComplexPlane"("Plane"=enum32{"Real", "Imaginary"}."Real", "Image"=w1031, "Image Pixels (float)"=w1014, "error in (no error)"=w1022) -> ("Image Out"=w1020:T3)  [unwired: 1 in, 1 out]
                n593 = call "IMAQ FFT"("Image Dst"=w1030, "Image Src"=w1020) -> ("error out"=w1019:errorcluster, "Image Dst Out"=w1018:T3)  [unwired: 2 in]
                n594 = local read "傅里叶最大值"() -> (w1013:dbl)
                n595 = call "IMAQ ComplexPlaneToArray"("error in (no error)"=w1019, "Plane"=T10."Magnitude", "Image"=w1018) -> ("Image Pixels (float)"=w1016:sgl[][])  [unwired: 2 in, 1 out]
                n596 = Add Array Elements(numeric array=w1016) -> (sum=w1011:sgl)
                "傅里叶求和" <- w1011
                n597 = Greater?(x=w1013, y=w1011) -> (0:w1025:bool)
                n598 = Select(t=w1013, s=w1025, f=w1011) -> (s? t:f=w1006:dbl)
                n599 = Multiply(x=w1006, y=0.98) -> (x*y=w1004:dbl)
                n600 = Less?(x=w1011, y=w1004) -> (x < y?=w1010:bool)
                n601 = local write "傅里叶最大值"(w1006) -> ()
                n602 = Multiply(x=w1006, y=0.9) -> (x*y=w1026:dbl)
                n603 = Multiply(x=w1006, y=0.95) -> (x*y=w1027:dbl)
                n604 = Less?(x=w1026, y=w1011) -> (x < y?=w1028:bool)
                n605 = Less?(x=w1011, y=w1027) -> (x < y?=w1029:bool)
                n606 = And(x=w1028, y=w1029) -> (x .and. y?=w1009:bool)
                n607 = Not(x=w1009) -> (.not. x?=w1008:bool)
                n608 = And(x=w1008, y=w1010) -> (x .and. y?=w1007:bool)
                n609 = case shown="真" w1007 {
                  tunnel: w1012 -> [_ w1033]
                  frame False {
                  }
                  frame True {
                    n610 = local write "傅里叶mp285下降步伐"(1.0 ("傅里叶最大值")) -> ()
                    n611 = call "SetZ_step.vi"("step"=12, "VISA资源名称"=w1033) -> ()  [unwired: 8 in, 2 out]
                  }
                }
              }
              frame #3 {
                n612 = local read "傅里叶数组"() -> (w1042:bool[])
                n613 = local read "已发送图像"() -> (w1035:bool)
                n614 = Insert Into Array(array=w1042, index=0 ("索引"), new element=w1037) -> (w1041:bool[])
                n615 = And Array Elements(Boolean array=w1042) -> (logical AND=w1046:bool)
                n616 = Or Array Elements(Boolean array=w1042) -> (logical OR=w1045:bool)
                n617 = And(x=w1037, y=w1046) -> (x .and. y?=w1039:bool)
                n618 = Not Or(1:w1045, 2:w1037) -> (0:w1044:bool)
                n619 = Delete From Array(array=w1041) -> (array with subset deleted=w1040:bool[])  [unwired: 2 in, 1 out]
                n620 = Or(x=w1039, y=w1035) -> (x .or. y?=w1036:bool)
                n621 = And(x=w1035, y=w1044) -> (x .and. y?=w1038:bool)
                n622 = local write "已发送图像"(w1036) -> ()
                n623 = local write "傅里叶数组"(w1040) -> ()
              }
              frame #4 {
                n624 = case shown="真" w1047 {
                  frame False {
                  }
                  frame True {
                    n625 = flat-sequence {
                      frame #0 {
                        n626 = One Button Dialog(message="没有细胞！！" ("消息")) -> ()  [unwired: 1 in, 1 out]
                        n627 = local write "没有细胞"(TRUE) -> ()
                      }
                      frame #1 {
                        w1051 = u16 0 items=["傅里叶初始", "傅里叶循环", "傅里叶暂停", "傅里叶结束"] ("傅里叶状态机")
                        n628 = local write "傅里叶状态机"(w1051) -> ()
                        n629 = local write "傅里叶"(FALSE ("傅里叶")) -> ()
                      }
                    }
                  }
                }
                n630 = case shown="真" w1048 {
                  frame False {
                  }
                  frame True {
                    w1054 = u16 2 items=["傅里叶初始", "傅里叶循环", "傅里叶暂停", "傅里叶结束"] ("傅里叶状态机")
                    n631 = local write "傅里叶状态机"(w1054) -> ()
                    n632 = local write "图像检测"(TRUE ("升Z轴找针")) -> ()
                    n633 = local write "图像检测到"(FALSE) -> ()
                  }
                }
              }
            }
          }
          frame 2 {
            n634 = local read "图像检测到"() -> (w1058:bool)
            n635 = local read "图像检测"() -> (w1056:bool)
            n636 = Not(x=w1056) -> (.not. x?=w1060:bool)
            n637 = And(x=w1058, y=w1060) -> (x .and. y?=w1059:bool)
            n638 = Or(x=w1056, y=w1058) -> (x .or. y?=w1057:bool)
            n639 = case shown="真" w1059 {
              frame False {
              }
              frame True {
                w1062 = u16 3 items=["傅里叶初始", "傅里叶循环", "傅里叶暂停", "傅里叶结束"] ("傅里叶状态机")
                n640 = local write "傅里叶状态机"(w1062) -> ()
              }
            }
            n641 = case shown="假" w1057 {
              frame False {
                w1061 = u16 1 items=["傅里叶初始", "傅里叶循环", "傅里叶暂停", "傅里叶结束"] ("傅里叶状态机")
                n642 = local write "傅里叶状态机"(w1061) -> ()
              }
              frame True {
              }
            }
          }
          frame 3 {
            n643 = flat-sequence {
              frame #0 {
                w1064 = u16 0 items=["傅里叶初始", "傅里叶循环", "傅里叶暂停", "傅里叶结束"] ("傅里叶状态机")
                n644 = local write "傅里叶"(FALSE ("傅里叶")) -> ()
                n645 = local write "傅里叶状态机"(w1064) -> ()
              }
              frame #1 {
                n646 = disable-structure shown="禁用" {
                  frame Disabled {
                    n647 = local write "开环移动针尖"(TRUE ("升Z轴找针")) -> ()
                  }
                  frame Enabled {
                  }
                }
              }
            }
          }
        }
      }
    }
    n648 = case shown="真" "自动接触" {
      tunnel: w874 -> [w1204 w1219]
      tunnel: [w1204 w1215] -> w898
      tunnel: w884 -> [_ w1206]
      frame False {
      }
      frame True {
        # "阈值"
        n649 = local read "校准的入液阻值"() -> (w1214:dbl)
        n650 = local read "阻值数组"() -> (w1225:dbl[])
        n651 = local read "自动接触初始"() -> (w1207:i32)
        n652 = Index Array(array=w1225, index=0 ("索引")) -> (element=w1218:dbl)
        n653 = Index Array(array=w1225, index=1 ("索引")) -> (element=w1223:dbl)
        n654 = Index Array(array=w1225, index=2 ("索引")) -> (element=w1222:dbl)
        n655 = Multiply(x=1.1, y=w1214) -> (x*y=w1212:dbl)
        n656 = Greater Or Equal?(x=w1218, y=w1223) -> (x >= y?=w1221:bool)
        n657 = Greater Or Equal?(x=w1223, y=w1222) -> (x >= y?=w1220:bool)
        n658 = Greater?(x=w1218, y=w1212) -> (0:w1217:bool)
        n659 = And(x=w1221, y=w1220) -> (x .and. y?=w1216:bool)
        n660 = And(x=w1217, y=w1216) -> (x .and. y?=w1208:bool)
        n661 = Boolean To (0,1)(Boolean=w1208) -> (0, 1=w1209:i16)
        n662 = Multiply(x=i16 10, y=w1209) -> (x*y=w1210:i16)
        n663 = Add(x=w1210, y=w1207) -> (x+y=w1205:i32)
        "自动接触状态" <- w1205
        n664 = case shown="0, 1, 默认" w1205 {
          tunnel: w1219 -> [w1229 w1274 w1324]
          tunnel: [w1228 w1275 w1324] -> w1215
          tunnel: w1206 -> [_ w1264 _]
          tunnel: w1205 -> [_ w1263 _]
          frame 10 {
            n665 = flat-sequence {
              tunnel: w1229 -> [w1235]
              tunnel: [w1234] -> w1228
              frame #0 {
                # "向下运动"
                n666 = local read "下降/向右"() -> (w1233:bool)
                n667 = local read "针下降次数"() -> (w1232:i32)
                n668 = case shown="真" w1233 {
                  tunnel: [-15.0 ("y") 0.0 ("X 2")] -> w1238
                  tunnel: [0.0 ("X 2") -15.0] -> w1237
                  tunnel: [0.0 ("Y 2") 0.0 ("Y 2")] -> w1236
                  frame False {
                  }
                  frame True {
                  }
                }
                n669 = Subtract(x=w1232, y=15) -> (x-y=w1231:i32)
                n670 = local write "针下降次数"(w1231) -> ()
                n671 = call "285_RelMove.vi"("VISA资源名称"=w1235, "Z 2"=w1238, "Y 2"=w1236, "X 2"=w1237) -> ("VISA resource name out 2"=w1234:refnum<visa-resource-name>)  [unwired: 2 in, 5 out]
              }
              frame #1 {
                n672 = Wait (ms)(milliseconds to wait=u32 3000 ("等待时间（毫秒）")) -> ()  [unwired: 1 out]
              }
              frame #2 {
                # "阈值"
                n673 = local read "校准的入液阻值"() -> (w1258:dbl)
                n674 = local read "阻值数组"() -> (w1256:dbl[])
                n675 = Index Array(array=w1256, index=0 ("索引")) -> (element=w1253:dbl)
                n676 = Index Array(array=w1256, index=1 ("索引")) -> (element=w1252:dbl)
                n677 = Index Array(array=w1256, index=2 ("索引")) -> (element=w1250:dbl)
                n678 = Multiply(x=1.08, y=w1258) -> (x*y=w1251:dbl)
                n679 = Greater?(x=w1251, y=w1252) -> (0:w1249:bool)
                n680 = Greater?(x=w1251, y=w1253) -> (0:w1248:bool)
                n681 = Greater?(x=w1251, y=w1250) -> (0:w1247:bool)
                n682 = Compound Arithmetic op=AND ("复合运算")(w1248, w1249, w1247) -> (w1246:bool)
                n683 = case shown="真" w1246 {
                  frame False {
                    n684 = local write "自动接触"(FALSE ("自动接触")) -> ()
                    n685 = One Button Dialog(message="堵针" ("消息")) -> ()  [unwired: 1 in, 1 out]
                  }
                  frame True {
                    n686 = local write "自动接触初始"(1) -> ()
                  }
                }
              }
            }
          }
          frame 0, 1, Default {
            # "向下运动"
            n687 = case shown="真" "下降/向右" {
              tunnel: ["下降步伐/um" 0.0 ("X 2")] -> w1272
              tunnel: [0.0 ("X 2") w1317] -> w1271
              tunnel: [0.0 ("Y 2") 0.0 ("Y 2")] -> w1270
              frame False {
              }
              frame True {
                n688 = local read "下降步伐/um"() -> (w1317:dbl)
              }
            }
            n689 = case shown="0" w1263 {
              tunnel: w1264 -> [w1276 _]
              frame 0 {
                n690 = flat-sequence {
                  tunnel: [w1281] -> w1278
                  tunnel: [w1280] -> w1277
                  tunnel: w1276 -> [w1279]
                  tunnel: w1278 -> [w1297]
                  tunnel: w1277 -> [w1296]
                  frame #0 {
                    n691 = VISA Flush I/O Buffer(VISA resource name=w1279) -> (VISA resource name out=w1289:refnum<visa-resource-name>, error out=w1290:errorcluster)  [unwired: 2 in]
                    n692 = Number To Decimal String(number=11 ("数字")) -> (decimal integer string=w1292:string)  [unwired: 1 in]
                    n693 = Concatenate Strings("C," ("字符串"), w1292, "\r") -> (w1294:string)
                    n694 = VISA Write ("VISA写入")(VISA resource name=w1289, write buffer=w1294, error in (no error)=w1290) -> (VISA resource name out=w1283:refnum<visa-resource-name>, error out=w1282:errorcluster)  [unwired: 1 out]
                    n695 = property class="Instr"(reference=w1283, error in=w1282) -> (reference out=w1284:refnum<visa-resource-name>, error out=w1285:errorcluster, "Serial Settings:Number of Bytes at Serial Port"=w1288:u32)
                    n696 = VISA Read(VISA resource name=w1284, byte count=w1288, error in (no error)=w1285) -> (VISA resource name out=w1286:refnum<visa-resource-name>, error out=w1287:errorcluster)  [unwired: 2 out]
                    n697 = VISA Flush I/O Buffer(VISA resource name=w1286, error in (no error)=w1287) -> (VISA resource name out=w1281:refnum<visa-resource-name>, error out=w1280:errorcluster)  [unwired: 1 in]
                  }
                  frame #1 {
                    n698 = disable-structure shown="禁用" {
                      disable-tunnel: w1297 -> [w1299 _]
                      disable-tunnel: w1296 -> [w1298 _]
                      frame Disabled {
                        n699 = Concatenate Strings("D" ("写入缓冲区"), "\r") -> (w1304:string)
                        n700 = VISA Write ("VISA写入")(VISA resource name=w1299, write buffer=w1304, error in (no error)=w1298) -> (VISA resource name out=w1309:refnum<visa-resource-name>, error out=w1307:errorcluster)  [unwired: 1 out]
                        n701 = property class="Instr"(reference=w1309, error in=w1307) -> (reference out=w1306:refnum<visa-resource-name>, error out=w1305:errorcluster, "Serial Settings:Number of Bytes at Serial Port"=w1308:u32)
                        n702 = VISA Read(VISA resource name=w1306, byte count=w1308, error in (no error)=w1305) -> (VISA resource name out=w1303:refnum<visa-resource-name>, error out=w1302:errorcluster)  [unwired: 2 out]
                        n703 = VISA Flush I/O Buffer(VISA resource name=w1303, error in (no error)=w1302) -> ()  [unwired: 1 in, 2 out]
                      }
                      frame Enabled {
                      }
                    }
                  }
                }
              }
              frame 1, Default {
              }
            }
            n704 = call "285_RelMove.vi"("VISA资源名称"=w1274, "Z 2"=w1272, "Y 2"=w1270, "X 2"=w1271) -> ("VISA resource name out 2"=w1275:refnum<visa-resource-name>)  [unwired: 2 in, 5 out]
            n705 = local read "针下降次数"() -> (w1269:i32)
            n706 = Add(x=w1269, y=1) -> (x+y=w1267:i32)
            n707 = Greater?(x=w1267, y=2000) -> (0:w1266:bool)
            n708 = case shown="真" w1266 {
              frame False {
              }
              frame True {
                n709 = local write "自动接触"(FALSE ("自动接触")) -> ()
                n710 = One Button Dialog(message="自动接触失败" ("消息")) -> ()  [unwired: 1 in, 1 out]
              }
            }
            n711 = local write "针下降次数"(w1267) -> ()
          }
          frame 11 {
            n712 = local write "自动接触"(FALSE) -> ()
            n713 = local write "自动封接"(TRUE) -> ()
            n714 = local write "自动接触初始"(0) -> ()
            n715 = local write "低负"(sgl -0.66 ("低负")) -> ()
            n716 = local write "针下降次数"(0) -> ()
            n717 = One Button Dialog(message="电极已接触细胞" ("消息")) -> ()  [unwired: 1 in, 1 out]
            n718 = Tick Count (ms)() -> (millisecond timer value=→"自动封接开始时间":u32)
          }
        }
      }
    }
    n719 = local read "针尖坐标"() -> (w881:sgl[])
    n720 = local read "目标坐标"() -> (w882:i32[])
    n721 = case shown="真" "开环移动针尖" {
      tunnel: w884 -> [_ _]
      tunnel: w874 -> [_ w923]
      tunnel: w882 -> [_ w922]
      tunnel: w881 -> [_ w921]
      frame False {
      }
      frame True {
        # "先上升大步伐，后上升小步伐"
        # "需要计算上升限制\n判断并结束"
        n722 = flat-sequence {
          tunnel: w923 -> [w936]
          tunnel: w922 -> [w935]
          tunnel: w921 -> [w934]
          frame #0 {
            n723 = Subtract(x=w935, y=w934) -> (x-y=w932:sgl[])
            n724 = Index Array(array=w932, index=1 ("索引")) -> (element=w929:sgl)
            n725 = Index Array(array=w932, index=0 ("索引")) -> (element=w930:sgl)
            n726 = Multiply(x=w929, y=sgl 0.119) -> (x*y=w928:sgl)
            n727 = Multiply(x=w930, y=sgl -0.123) -> (x*y=w927:sgl)
            n728 = call "285_RelMove.vi"("VISA资源名称"=w936, "Z 2"=0 ("y"), "Y 2"=w928, "X 2"=w927) -> ()  [unwired: 2 in, 6 out]
          }
          frame #1 {
            n729 = Wait (ms)(milliseconds to wait=u32 1000 ("等待时间（毫秒）")) -> ()  [unwired: 1 out]
          }
          frame #2 {
            w938 = u16 1 items=["高正压", "低正压", "大气压", "低负压", "高负压"] ("气压选择")
            n730 = disable-structure shown="禁用" {
              frame Disabled {
                n731 = local write "自动接触"(TRUE ("针尖自动移动 2")) -> ()
              }
              frame Enabled {
              }
            }
            n732 = local read "Resistance(MΩ)"() -> (→"校准的入液阻值":dbl)
            n733 = local write "自动接触初始"(0 ("自动接触初始")) -> ()
            n734 = local write "开环移动针尖"(FALSE ("升Z轴找针")) -> ()
            n735 = local write "气压选择"(w938) -> ()
          }
        }
      }
    }
    n736 = case shown="真" "没有细胞" {
      frame False {
      }
      frame True {
        # "目标坐标"
        n737 = property on="Image" class="ImageControl"() -> ("ROI"=w909:T11)  [unwired: 2 in, 2 out]
        n738 = Unbundle(w909) -> ("Global Rectangle"=w907:i32[])  [unwired: 1 out]
        n739 = Array Subset(array=w907, index=0 ("索引"), length=2 ("长度")) -> (→"目标坐标":i32[])
      }
    }
    n740 = case shown="真" "保存数据" {
      tunnel: w898 -> [w1141 w1157]
      tunnel: [w1132 w1157] -> w891
      tunnel: w896 -> [w1134 w1156]
      tunnel: w895 -> [w1130 _]
      tunnel: [w1133 w1156] -> w892
      tunnel: w894 -> [w1128 _]
      frame True {
        w1124 = "\t"
        n741 = local read "Resistance(MΩ)"() -> (w1131:dbl)
        n742 = call "285_GetPos.vi"("VISA资源名称"=w1141) -> ("Z"=w1136:dbl, "Y"=w1138:dbl, "X"=w1140:dbl, "VISA资源名称输出"=w1132:refnum<visa-resource-name>)  [unwired: 5 in, 2 out]
        n743 = Quotient & Remainder(x=w1128, y=100) -> (x-y*floor(x/y)=w1126:i32)  [unwired: 1 out]
        n744 = Get Date/Time String(want seconds? (F)=TRUE ("需要秒？(F)")) -> (time string=w1122:string)  [unwired: 2 in, 1 out]
        n745 = Number To Fractional String(number=w1138) -> (F-format string=w1137:string)  [unwired: 3 in]
        n746 = Number To Decimal String(number=w1128) -> (decimal integer string=w1129:string)  [unwired: 1 in]
        n747 = Number To Fractional String(number=w1140) -> (F-format string=w1139:string)  [unwired: 3 in]
        n748 = Number To Fractional String(number=w1136) -> (F-format string=w1135:string)  [unwired: 3 in]
        n749 = Number To Fractional String(number=w1131) -> (F-format string=w1147:string)  [unwired: 3 in]
        n750 = Equal?(x=w1126, y=0) -> (x = y?=w1121:bool)
        n751 = case shown="真" w1121 {
          tunnel: w1130 -> [_ w1151]
          tunnel: w1129 -> [_ w1149]
          frame False {
          }
          frame True {
            n752 = Concatenate Strings("图像" ("字符串"), w1149, ".bmp" ("字符串")) -> (w1153:string)
            n753 = local read "Image"() -> (w1150:T3)
            n754 = Build Path(base path=w1151, name or relative path=w1153) -> (appended path=w1155:path)
            n755 = call-poly "IMAQ Write File 2"("File Path"=w1155, "Image"=w1150) -> ()  [unwired: 8 in, 2 out]
          }
        }
        n756 = Concatenate Strings(w1122, w1124, w1129, w1124, w1124, "X轴：" ("字符串"), w1139, w1124, "Y轴：" ("字符串"), w1137, w1124, "Z轴：" ("字符串"), w1135, w1124, "阻值：" ("字符串"), w1147, "\n") -> (w1142:string)
        n757 = Write to Text File(file (use dialog)=w1134, text=w1142) -> (refnum out=w1133:refnum<file>)  [unwired: 2 in, 2 out]
      }
      frame False {
      }
    }
  }
  n758 = call "IMAQ Dispose"("Image"=w17) -> ()  [unwired: 5 in, 1 out]
  n759 = call "IMAQ Dispose"("Image"=w18) -> ()  [unwired: 5 in, 1 out]
  n760 = Close File(refnum=w46) -> ()  [unwired: 1 in, 2 out]
  n761 = call "285_Update.vi"("VISA资源名称"=w26) -> ("VISA资源名称 2"=w62:refnum<visa-resource-name>)  [unwired: 9 in, 1 out]
  n762 = VISA Close(VISA resource name=w62) -> ()  [unwired: 1 in, 1 out]
  n763 = disable-structure shown="禁用" {
    frame Disabled {
      n764 = call "285_Update.vi"() -> ("VISA资源名称 2"=w1326:refnum<visa-resource-name>)  [unwired: 10 in, 1 out]
      n765 = VISA Close(VISA resource name=w1326) -> ()  [unwired: 1 in, 1 out]
    }
    frame Enabled {
    }
  }
